vi "Write SerDes GPIO Bank Output Enable.vi"(0 "gpio bank output enable":T2, 2 "serdes id":T1=enum."SI 0 Deserializer") -> (4 "serdes id valid":bool)   [LabVIEW 2020, in "GettingStarted_Common_148X_FPGA.lvlib"]
uses:
  GettingStarted_Common_148X_FPGA.lvlib
  <instrlib>/FlexRIO/CSI-2/v2/FPGA/Types/GPIO Bank.ctl
  Types/SerDes Identifier.ctl
  <vilib>/eio/EIONode/EIONode.xnode
  <vilib>/rvi/eio/common/nirviEmuTemplateMethod_errors.vi
  <instrlib>/_niInstr/Basic Elements/v1/FPGA/niInstr Basic Elements v1 FPGA.lvlib
  <instrlib>/FlexRIO/CSI-2/v2/FPGA/NI CSI-2 API FPGA v2.lvlib
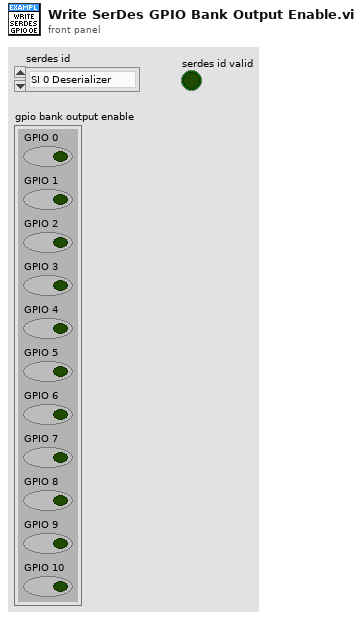
[diagram p1: front panel]
types:
  T1 = typedef "GettingStarted_Common_148X_FPGA.lvlib/SerDes Identifier.ctl" = enum8{"None", "SI 0 Deserializer", "SI 1 Deserializer", "SI 2 Deserializer", "SI 3 Deserializer", "SI 4 Deserializer", "SI 5 Deserializer", "SI 6 Deserializer", "SI 7 Deserializer", "SO 0 Serializer", "SO 1 Serializer", "SO 2 Serializer", "SO 3 Serializer", "SO 4 Serializer", "SO 5 Serializer", "SO 6 Serializer", "SO 7 Serializer", "SI 0 SI 1 Deserializer", "SI 2 SI 3 Deserializer", "SI 4 SI 5 Deserializer", "SI 6 SI 7 Deserializer"}
  T2 = typedef "NI CSI-2 API FPGA v2.lvlib/GPIO Bank.ctl" = cluster{"GPIO 0":bool, "GPIO 1":bool, "GPIO 2":bool, "GPIO 3":bool, "GPIO 4":bool, "GPIO 5":bool, "GPIO 6":bool, "GPIO 7":bool, "GPIO 8":bool, "GPIO 9":bool, "GPIO 10":bool}
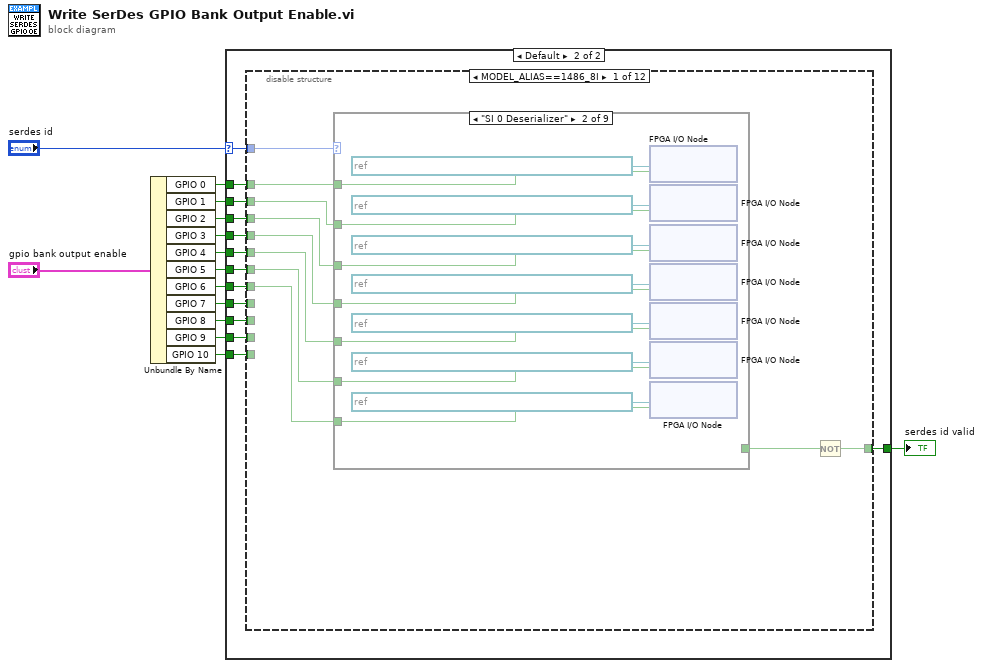
[diagram p0: block diagram]
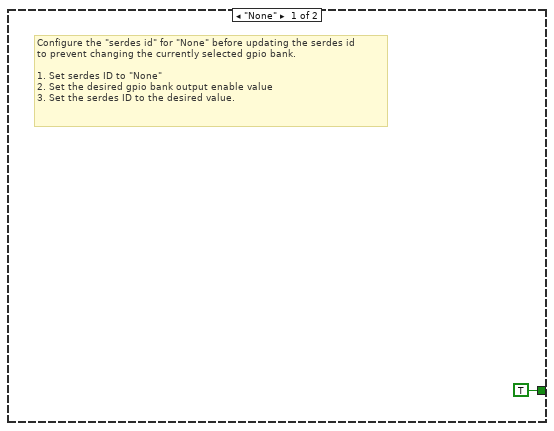
[diagram p2: hidden frame]
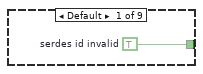
[diagram p3: hidden frame]
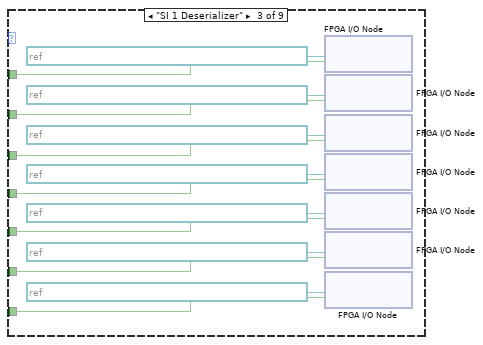
[diagram p4: hidden frame]
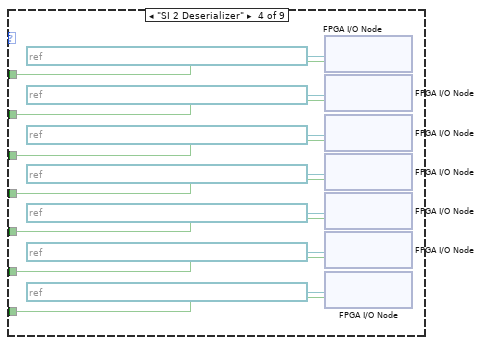
[diagram p5: hidden frame]
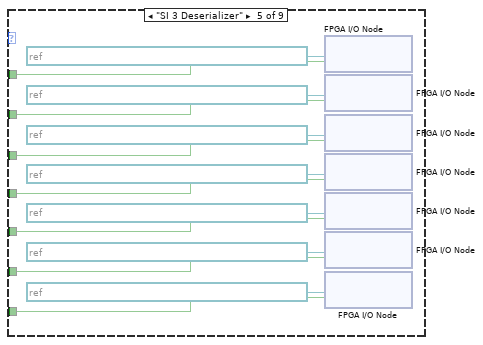
[diagram p6: hidden frame]
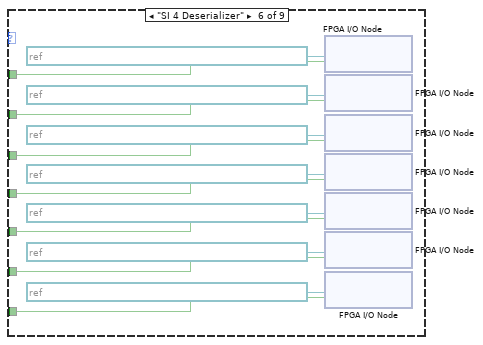
[diagram p7: hidden frame]
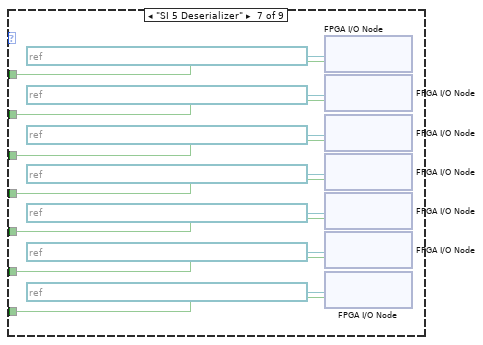
[diagram p8: hidden frame]
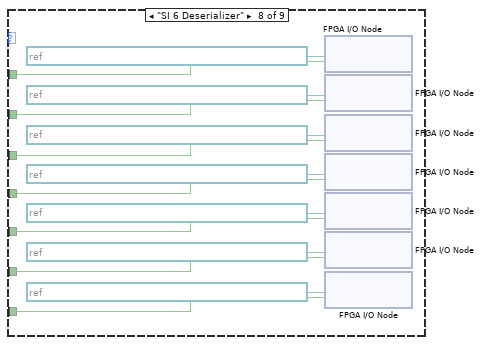
[diagram p9: hidden frame]
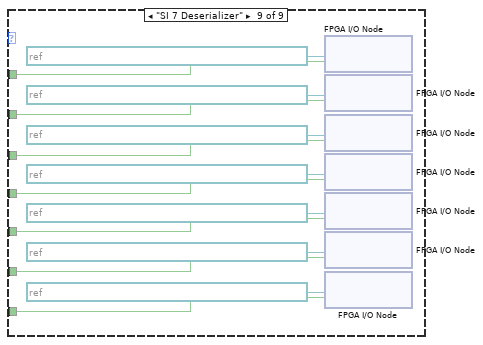
[diagram p10: hidden frame]
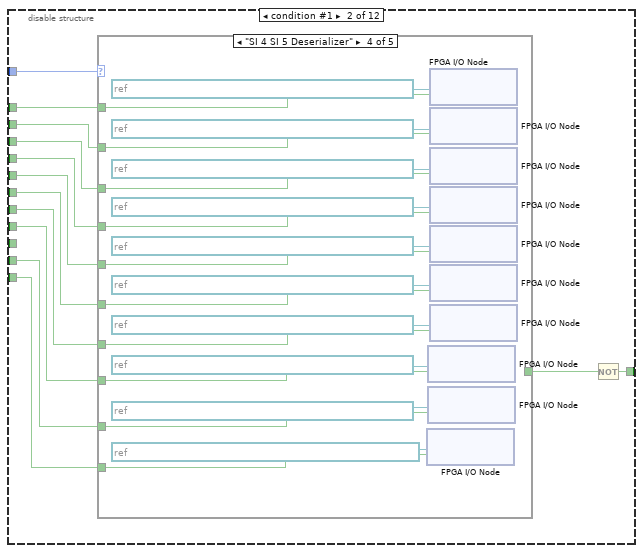
[diagram p11: hidden frame]
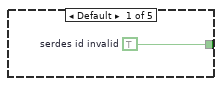
[diagram p12: hidden frame]
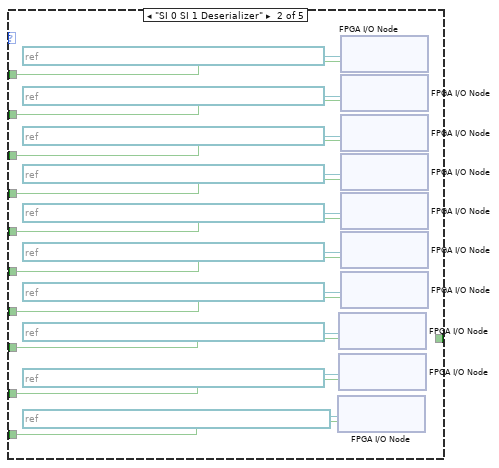
[diagram p13: hidden frame]
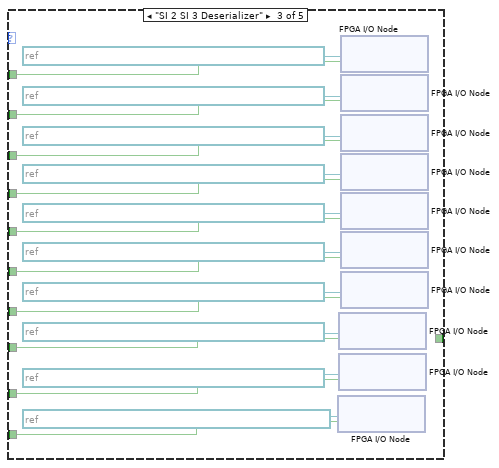
[diagram p14: hidden frame]
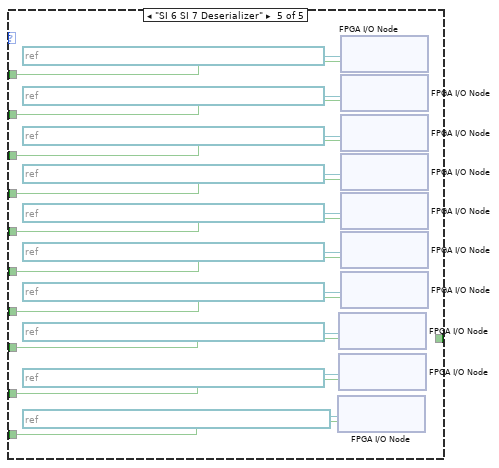
[diagram p15: hidden frame]
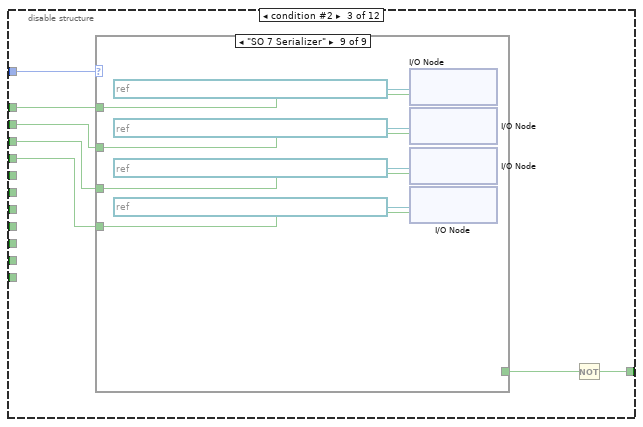
[diagram p16: hidden frame]
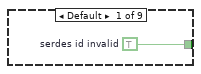
[diagram p17: hidden frame]
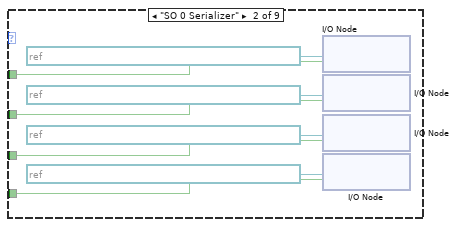
[diagram p18: hidden frame]
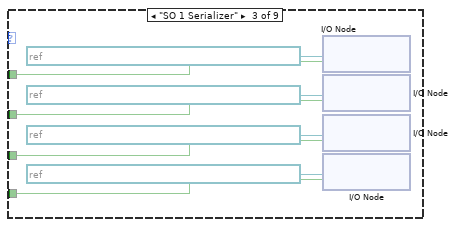
[diagram p19: hidden frame]
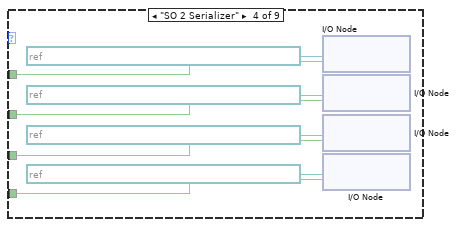
[diagram p20: hidden frame]
diagram:
  n1 = Unbundle By Name("gpio bank output enable") -> ("GPIO 0"=w2:bool, "GPIO 1"=w3:bool, "GPIO 2"=w4:bool, "GPIO 3"=w5:bool, "GPIO 4"=w6:bool, "GPIO 5"=w7:bool, "GPIO 6"=w8:bool, "GPIO 7"=w9:bool, "GPIO 8"=w10:bool, "GPIO 9"=w11:bool, "GPIO 10"=w12:bool)
  n2 = case shown="Default" "serdes id" {
    selector: "serdes id" -> [_ w16]
    tunnel: [TRUE w28] -> w13
    tunnel: w12 -> [_ w27]
    tunnel: w11 -> [_ w26]
    tunnel: w10 -> [_ w25]
    tunnel: w9 -> [_ w24]
    tunnel: w8 -> [_ w23]
    tunnel: w7 -> [_ w22]
    tunnel: w6 -> [_ w21]
    tunnel: w5 -> [_ w20]
    tunnel: w4 -> [_ w19]
    tunnel: w3 -> [_ w18]
    tunnel: w2 -> [_ w17]
    frame "None" {
      # "Configure the \"serdes id\" for \"None\" before updating the serdes id\nto prevent changing the currently selected gpio bank.\n\n1. Set serdes ID to \"None\" \n2. Set the desired gpio bank output enable value \n3. Set the serdes ID to the desired value."
    }
    frame Default {
      n3 = disable-structure shown="MODEL_ALIAS==1486_8I" {
        disable-tunnel: w16 -> [w38 w163 w252 w327 w429 w556 w643 w689 w795 w858 w993 _]
        disable-tunnel: w17 -> [w37 w162 w251 w326 w428 w555 w642 w688 w794 w857 w992 _]
        disable-tunnel: w18 -> [w36 w161 w250 w325 w427 w554 w641 _ _ w856 w991 _]
        disable-tunnel: w19 -> [w35 w160 w249 w324 w426 w553 w640 _ _ w855 w990 _]
        disable-tunnel: w20 -> [w34 w159 w248 w323 w425 w552 w639 w687 w793 w854 w989 _]
        disable-tunnel: w21 -> [w33 w158 _ w322 w424 w551 w638 w686 w792 w853 w988 _]
        disable-tunnel: w22 -> [w32 w157 _ w321 w423 w550 w637 _ _ w852 w987 _]
        disable-tunnel: w23 -> [w31 w156 _ w320 w422 w549 w636 w685 w791 w851 w986 _]
        disable-tunnel: w24 -> [_ w155 _ _ w419 w546 w633 w682 w788 w848 w983 _]
        disable-tunnel: w25 -> [_ _ _ _ _ w545 w632 w681 w787 w847 w982 _]
        disable-tunnel: w26 -> [_ w154 _ _ w418 w544 w631 _ _ w846 w981 _]
        disable-tunnel: w27 -> [_ w153 _ _ w417 w543 w630 _ _ w845 w980 _]
        disable-tunnel: [w29 w164 w246 w318 w420 w547 w634 w683 w789 w849 w984 _] -> w28
        frame condition #0 {
          n4 = case shown="\"SI 0 Deserializer\"" w38 {
            tunnel: w37 -> [_ w46 w60 w74 w88 w102 w116 w130 w144]
            tunnel: w36 -> [_ w45 w59 w73 w87 w101 w115 w129 w143]
            tunnel: w35 -> [_ w44 w58 w72 w86 w100 w114 w128 w142]
            tunnel: w34 -> [_ w43 w57 w71 w85 w99 w113 w127 w141]
            tunnel: w33 -> [_ w42 w56 w70 w84 w98 w112 w126 w140]
            tunnel: w32 -> [_ w41 w55 w69 w83 w97 w111 w125 w139]
            tunnel: w31 -> [_ w40 w54 w68 w82 w96 w110 w124 w138]
            tunnel: [w39 _ _ _ _ _ _ _ _] -> w30
            frame Default {
              w39 = TRUE  # serdes id invalid
            }
            frame "SI 0 Deserializer" {
              n5 = xnode "FPGA I/O Node"("I/O Item"=w46, "FPGA I/O In"=refnum<k21> "IO Socket\\SI 0 Deserializer GPIO 0 Output Enable") -> ()  [unwired: 1 out]
              n6 = xnode "FPGA I/O Node"("I/O Item"=w45, "FPGA I/O In"=refnum<k21> "IO Socket\\SI 0 Deserializer GPIO 1 Output Enable") -> ()  [unwired: 1 out]
              n7 = xnode "FPGA I/O Node"("I/O Item"=w44, "FPGA I/O In"=refnum<k21> "IO Socket\\SI 0 Deserializer GPIO 2 Output Enable") -> ()  [unwired: 1 out]
              n8 = xnode "FPGA I/O Node"("I/O Item"=w43, "FPGA I/O In"=refnum<k21> "IO Socket\\SI 0 Deserializer GPIO 3 Output Enable") -> ()  [unwired: 1 out]
              n9 = xnode "FPGA I/O Node"("I/O Item"=w42, "FPGA I/O In"=refnum<k21> "IO Socket\\SI 0 Deserializer GPIO 4 Output Enable") -> ()  [unwired: 1 out]
              n10 = xnode "FPGA I/O Node"("I/O Item"=w41, "FPGA I/O In"=refnum<k21> "IO Socket\\SI 0 Deserializer GPIO 5 Output Enable") -> ()  [unwired: 1 out]
              n11 = xnode "FPGA I/O Node"("I/O Item"=w40, "FPGA I/O In"=refnum<k21> "IO Socket\\SI 0 Deserializer GPIO 6 Output Enable") -> ()  [unwired: 1 out]
            }
            frame "SI 1 Deserializer" {
              n12 = xnode "FPGA I/O Node"("I/O Item"=w60, "FPGA I/O In"=refnum<k21> "IO Socket\\SI 1 Deserializer GPIO 0 Output Enable") -> ()  [unwired: 1 out]
              n13 = xnode "FPGA I/O Node"("I/O Item"=w59, "FPGA I/O In"=refnum<k21> "IO Socket\\SI 1 Deserializer GPIO 1 Output Enable") -> ()  [unwired: 1 out]
              n14 = xnode "FPGA I/O Node"("I/O Item"=w58, "FPGA I/O In"=refnum<k21> "IO Socket\\SI 1 Deserializer GPIO 2 Output Enable") -> ()  [unwired: 1 out]
              n15 = xnode "FPGA I/O Node"("I/O Item"=w57, "FPGA I/O In"=refnum<k21> "IO Socket\\SI 1 Deserializer GPIO 3 Output Enable") -> ()  [unwired: 1 out]
              n16 = xnode "FPGA I/O Node"("I/O Item"=w56, "FPGA I/O In"=refnum<k21> "IO Socket\\SI 1 Deserializer GPIO 4 Output Enable") -> ()  [unwired: 1 out]
              n17 = xnode "FPGA I/O Node"("I/O Item"=w55, "FPGA I/O In"=refnum<k21> "IO Socket\\SI 1 Deserializer GPIO 5 Output Enable") -> ()  [unwired: 1 out]
              n18 = xnode "FPGA I/O Node"("I/O Item"=w54, "FPGA I/O In"=refnum<k21> "IO Socket\\SI 1 Deserializer GPIO 6 Output Enable") -> ()  [unwired: 1 out]
            }
            frame "SI 2 Deserializer" {
              n19 = xnode "FPGA I/O Node"("I/O Item"=w74, "FPGA I/O In"=refnum<k21> "IO Socket\\SI 2 Deserializer GPIO 0 Output Enable") -> ()  [unwired: 1 out]
              n20 = xnode "FPGA I/O Node"("I/O Item"=w73, "FPGA I/O In"=refnum<k21> "IO Socket\\SI 2 Deserializer GPIO 1 Output Enable") -> ()  [unwired: 1 out]
              n21 = xnode "FPGA I/O Node"("I/O Item"=w72, "FPGA I/O In"=refnum<k21> "IO Socket\\SI 2 Deserializer GPIO 2 Output Enable") -> ()  [unwired: 1 out]
              n22 = xnode "FPGA I/O Node"("I/O Item"=w71, "FPGA I/O In"=refnum<k21> "IO Socket\\SI 2 Deserializer GPIO 3 Output Enable") -> ()  [unwired: 1 out]
              n23 = xnode "FPGA I/O Node"("I/O Item"=w70, "FPGA I/O In"=refnum<k21> "IO Socket\\SI 2 Deserializer GPIO 4 Output Enable") -> ()  [unwired: 1 out]
              n24 = xnode "FPGA I/O Node"("I/O Item"=w69, "FPGA I/O In"=refnum<k21> "IO Socket\\SI 2 Deserializer GPIO 5 Output Enable") -> ()  [unwired: 1 out]
              n25 = xnode "FPGA I/O Node"("I/O Item"=w68, "FPGA I/O In"=refnum<k21> "IO Socket\\SI 2 Deserializer GPIO 6 Output Enable") -> ()  [unwired: 1 out]
            }
            frame "SI 3 Deserializer" {
              n26 = xnode "FPGA I/O Node"("I/O Item"=w88, "FPGA I/O In"=refnum<k21> "IO Socket\\SI 3 Deserializer GPIO 0 Output Enable") -> ()  [unwired: 1 out]
              n27 = xnode "FPGA I/O Node"("I/O Item"=w87, "FPGA I/O In"=refnum<k21> "IO Socket\\SI 3 Deserializer GPIO 1 Output Enable") -> ()  [unwired: 1 out]
              n28 = xnode "FPGA I/O Node"("I/O Item"=w86, "FPGA I/O In"=refnum<k21> "IO Socket\\SI 3 Deserializer GPIO 2 Output Enable") -> ()  [unwired: 1 out]
              n29 = xnode "FPGA I/O Node"("I/O Item"=w85, "FPGA I/O In"=refnum<k21> "IO Socket\\SI 3 Deserializer GPIO 3 Output Enable") -> ()  [unwired: 1 out]
              n30 = xnode "FPGA I/O Node"("I/O Item"=w84, "FPGA I/O In"=refnum<k21> "IO Socket\\SI 3 Deserializer GPIO 4 Output Enable") -> ()  [unwired: 1 out]
              n31 = xnode "FPGA I/O Node"("I/O Item"=w83, "FPGA I/O In"=refnum<k21> "IO Socket\\SI 3 Deserializer GPIO 5 Output Enable") -> ()  [unwired: 1 out]
              n32 = xnode "FPGA I/O Node"("I/O Item"=w82, "FPGA I/O In"=refnum<k21> "IO Socket\\SI 3 Deserializer GPIO 6 Output Enable") -> ()  [unwired: 1 out]
            }
            frame "SI 4 Deserializer" {
              n33 = xnode "FPGA I/O Node"("I/O Item"=w102, "FPGA I/O In"=refnum<k21> "IO Socket\\SI 4 Deserializer GPIO 0 Output Enable") -> ()  [unwired: 1 out]
              n34 = xnode "FPGA I/O Node"("I/O Item"=w101, "FPGA I/O In"=refnum<k21> "IO Socket\\SI 4 Deserializer GPIO 1 Output Enable") -> ()  [unwired: 1 out]
              n35 = xnode "FPGA I/O Node"("I/O Item"=w100, "FPGA I/O In"=refnum<k21> "IO Socket\\SI 4 Deserializer GPIO 2 Output Enable") -> ()  [unwired: 1 out]
              n36 = xnode "FPGA I/O Node"("I/O Item"=w99, "FPGA I/O In"=refnum<k21> "IO Socket\\SI 4 Deserializer GPIO 3 Output Enable") -> ()  [unwired: 1 out]
              n37 = xnode "FPGA I/O Node"("I/O Item"=w98, "FPGA I/O In"=refnum<k21> "IO Socket\\SI 4 Deserializer GPIO 4 Output Enable") -> ()  [unwired: 1 out]
              n38 = xnode "FPGA I/O Node"("I/O Item"=w97, "FPGA I/O In"=refnum<k21> "IO Socket\\SI 4 Deserializer GPIO 5 Output Enable") -> ()  [unwired: 1 out]
              n39 = xnode "FPGA I/O Node"("I/O Item"=w96, "FPGA I/O In"=refnum<k21> "IO Socket\\SI 4 Deserializer GPIO 6 Output Enable") -> ()  [unwired: 1 out]
            }
            frame "SI 5 Deserializer" {
              n40 = xnode "FPGA I/O Node"("I/O Item"=w116, "FPGA I/O In"=refnum<k21> "IO Socket\\SI 5 Deserializer GPIO 0 Output Enable") -> ()  [unwired: 1 out]
              n41 = xnode "FPGA I/O Node"("I/O Item"=w115, "FPGA I/O In"=refnum<k21> "IO Socket\\SI 5 Deserializer GPIO 1 Output Enable") -> ()  [unwired: 1 out]
              n42 = xnode "FPGA I/O Node"("I/O Item"=w114, "FPGA I/O In"=refnum<k21> "IO Socket\\SI 5 Deserializer GPIO 2 Output Enable") -> ()  [unwired: 1 out]
              n43 = xnode "FPGA I/O Node"("I/O Item"=w113, "FPGA I/O In"=refnum<k21> "IO Socket\\SI 5 Deserializer GPIO 3 Output Enable") -> ()  [unwired: 1 out]
              n44 = xnode "FPGA I/O Node"("I/O Item"=w112, "FPGA I/O In"=refnum<k21> "IO Socket\\SI 5 Deserializer GPIO 4 Output Enable") -> ()  [unwired: 1 out]
              n45 = xnode "FPGA I/O Node"("I/O Item"=w111, "FPGA I/O In"=refnum<k21> "IO Socket\\SI 5 Deserializer GPIO 5 Output Enable") -> ()  [unwired: 1 out]
              n46 = xnode "FPGA I/O Node"("I/O Item"=w110, "FPGA I/O In"=refnum<k21> "IO Socket\\SI 5 Deserializer GPIO 6 Output Enable") -> ()  [unwired: 1 out]
            }
            frame "SI 6 Deserializer" {
              n47 = xnode "FPGA I/O Node"("I/O Item"=w130, "FPGA I/O In"=refnum<k21> "IO Socket\\SI 6 Deserializer GPIO 0 Output Enable") -> ()  [unwired: 1 out]
              n48 = xnode "FPGA I/O Node"("I/O Item"=w129, "FPGA I/O In"=refnum<k21> "IO Socket\\SI 6 Deserializer GPIO 1 Output Enable") -> ()  [unwired: 1 out]
              n49 = xnode "FPGA I/O Node"("I/O Item"=w128, "FPGA I/O In"=refnum<k21> "IO Socket\\SI 6 Deserializer GPIO 2 Output Enable") -> ()  [unwired: 1 out]
              n50 = xnode "FPGA I/O Node"("I/O Item"=w127, "FPGA I/O In"=refnum<k21> "IO Socket\\SI 6 Deserializer GPIO 3 Output Enable") -> ()  [unwired: 1 out]
              n51 = xnode "FPGA I/O Node"("I/O Item"=w126, "FPGA I/O In"=refnum<k21> "IO Socket\\SI 6 Deserializer GPIO 4 Output Enable") -> ()  [unwired: 1 out]
              n52 = xnode "FPGA I/O Node"("I/O Item"=w125, "FPGA I/O In"=refnum<k21> "IO Socket\\SI 6 Deserializer GPIO 5 Output Enable") -> ()  [unwired: 1 out]
              n53 = xnode "FPGA I/O Node"("I/O Item"=w124, "FPGA I/O In"=refnum<k21> "IO Socket\\SI 6 Deserializer GPIO 6 Output Enable") -> ()  [unwired: 1 out]
            }
            frame "SI 7 Deserializer" {
              n54 = xnode "FPGA I/O Node"("I/O Item"=w144, "FPGA I/O In"=refnum<k21> "IO Socket\\SI 7 Deserializer GPIO 0 Output Enable") -> ()  [unwired: 1 out]
              n55 = xnode "FPGA I/O Node"("I/O Item"=w143, "FPGA I/O In"=refnum<k21> "IO Socket\\SI 7 Deserializer GPIO 1 Output Enable") -> ()  [unwired: 1 out]
              n56 = xnode "FPGA I/O Node"("I/O Item"=w142, "FPGA I/O In"=refnum<k21> "IO Socket\\SI 7 Deserializer GPIO 2 Output Enable") -> ()  [unwired: 1 out]
              n57 = xnode "FPGA I/O Node"("I/O Item"=w141, "FPGA I/O In"=refnum<k21> "IO Socket\\SI 7 Deserializer GPIO 3 Output Enable") -> ()  [unwired: 1 out]
              n58 = xnode "FPGA I/O Node"("I/O Item"=w140, "FPGA I/O In"=refnum<k21> "IO Socket\\SI 7 Deserializer GPIO 4 Output Enable") -> ()  [unwired: 1 out]
              n59 = xnode "FPGA I/O Node"("I/O Item"=w139, "FPGA I/O In"=refnum<k21> "IO Socket\\SI 7 Deserializer GPIO 5 Output Enable") -> ()  [unwired: 1 out]
              n60 = xnode "FPGA I/O Node"("I/O Item"=w138, "FPGA I/O In"=refnum<k21> "IO Socket\\SI 7 Deserializer GPIO 6 Output Enable") -> ()  [unwired: 1 out]
            }
          }
          n61 = Not(x=w30) -> (.not. x?=w29:bool)
        }
        frame condition #1 {
          n62 = case shown="\"SI 4 SI 5 Deserializer\"" w163 {
            tunnel: w162 -> [_ w185 w205 w225 w245]
            tunnel: w161 -> [_ w184 w204 w224 w244]
            tunnel: w160 -> [_ w183 w203 w223 w243]
            tunnel: w159 -> [_ w182 w202 w222 w242]
            tunnel: w158 -> [_ w181 w201 w221 w241]
            tunnel: w157 -> [_ w180 w200 w220 w240]
            tunnel: w156 -> [_ w179 w199 w219 w239]
            tunnel: [w165 _ _ _ _] -> w152
            tunnel: w155 -> [_ w168 w188 w208 w228]
            tunnel: w154 -> [_ w167 w187 w207 w227]
            tunnel: w153 -> [_ w166 w186 w206 w226]
            frame Default {
              w165 = TRUE  # serdes id invalid
            }
            frame "SI 0 SI 1 Deserializer" {
              n63 = xnode "FPGA I/O Node"("I/O Item"=w166, "FPGA I/O In"=refnum<k21> "IO Socket\\SI 0 SI 1 Deserializer GPIO 10 Output Enable") -> ()  [unwired: 1 out]
              n64 = xnode "FPGA I/O Node"("I/O Item"=w168, "FPGA I/O In"=refnum<k21> "IO Socket\\SI 0 SI 1 Deserializer GPIO 7 Output Enable") -> ()  [unwired: 1 out]
              n65 = xnode "FPGA I/O Node"("I/O Item"=w167, "FPGA I/O In"=refnum<k21> "IO Socket\\SI 0 SI 1 Deserializer GPIO 9 Output Enable") -> ()  [unwired: 1 out]
              n66 = xnode "FPGA I/O Node"("I/O Item"=w185, "FPGA I/O In"=refnum<k21> "IO Socket\\SI 0 SI 1 Deserializer GPIO 0 Output Enable") -> ()  [unwired: 1 out]
              n67 = xnode "FPGA I/O Node"("I/O Item"=w184, "FPGA I/O In"=refnum<k21> "IO Socket\\SI 0 SI 1 Deserializer GPIO 1 Output Enable") -> ()  [unwired: 1 out]
              n68 = xnode "FPGA I/O Node"("I/O Item"=w183, "FPGA I/O In"=refnum<k21> "IO Socket\\SI 0 SI 1 Deserializer GPIO 2 Output Enable") -> ()  [unwired: 1 out]
              n69 = xnode "FPGA I/O Node"("I/O Item"=w182, "FPGA I/O In"=refnum<k21> "IO Socket\\SI 0 SI 1 Deserializer GPIO 3 Output Enable") -> ()  [unwired: 1 out]
              n70 = xnode "FPGA I/O Node"("I/O Item"=w181, "FPGA I/O In"=refnum<k21> "IO Socket\\SI 0 SI 1 Deserializer GPIO 4 Output Enable") -> ()  [unwired: 1 out]
              n71 = xnode "FPGA I/O Node"("I/O Item"=w180, "FPGA I/O In"=refnum<k21> "IO Socket\\SI 0 SI 1 Deserializer GPIO 5 Output Enable") -> ()  [unwired: 1 out]
              n72 = xnode "FPGA I/O Node"("I/O Item"=w179, "FPGA I/O In"=refnum<k21> "IO Socket\\SI 0 SI 1 Deserializer GPIO 6 Output Enable") -> ()  [unwired: 1 out]
            }
            frame "SI 2 SI 3 Deserializer" {
              n73 = xnode "FPGA I/O Node"("I/O Item"=w186, "FPGA I/O In"=refnum<k21> "IO Socket\\SI 2 SI 3 Deserializer GPIO 10 Output Enable") -> ()  [unwired: 1 out]
              n74 = xnode "FPGA I/O Node"("I/O Item"=w188, "FPGA I/O In"=refnum<k21> "IO Socket\\SI 2 SI 3 Deserializer GPIO 7 Output Enable") -> ()  [unwired: 1 out]
              n75 = xnode "FPGA I/O Node"("I/O Item"=w187, "FPGA I/O In"=refnum<k21> "IO Socket\\SI 2 SI 3 Deserializer GPIO 9 Output Enable") -> ()  [unwired: 1 out]
              n76 = xnode "FPGA I/O Node"("I/O Item"=w205, "FPGA I/O In"=refnum<k21> "IO Socket\\SI 2 SI 3 Deserializer GPIO 0 Output Enable") -> ()  [unwired: 1 out]
              n77 = xnode "FPGA I/O Node"("I/O Item"=w204, "FPGA I/O In"=refnum<k21> "IO Socket\\SI 2 SI 3 Deserializer GPIO 1 Output Enable") -> ()  [unwired: 1 out]
              n78 = xnode "FPGA I/O Node"("I/O Item"=w203, "FPGA I/O In"=refnum<k21> "IO Socket\\SI 2 SI 3 Deserializer GPIO 2 Output Enable") -> ()  [unwired: 1 out]
              n79 = xnode "FPGA I/O Node"("I/O Item"=w202, "FPGA I/O In"=refnum<k21> "IO Socket\\SI 2 SI 3 Deserializer GPIO 3 Output Enable") -> ()  [unwired: 1 out]
              n80 = xnode "FPGA I/O Node"("I/O Item"=w201, "FPGA I/O In"=refnum<k21> "IO Socket\\SI 2 SI 3 Deserializer GPIO 4 Output Enable") -> ()  [unwired: 1 out]
              n81 = xnode "FPGA I/O Node"("I/O Item"=w200, "FPGA I/O In"=refnum<k21> "IO Socket\\SI 2 SI 3 Deserializer GPIO 5 Output Enable") -> ()  [unwired: 1 out]
              n82 = xnode "FPGA I/O Node"("I/O Item"=w199, "FPGA I/O In"=refnum<k21> "IO Socket\\SI 2 SI 3 Deserializer GPIO 6 Output Enable") -> ()  [unwired: 1 out]
            }
            frame "SI 4 SI 5 Deserializer" {
              n83 = xnode "FPGA I/O Node"("I/O Item"=w206, "FPGA I/O In"=refnum<k21> "IO Socket\\SI 4 SI 5 Deserializer GPIO 10 Output Enable") -> ()  [unwired: 1 out]
              n84 = xnode "FPGA I/O Node"("I/O Item"=w208, "FPGA I/O In"=refnum<k21> "IO Socket\\SI 4 SI 5 Deserializer GPIO 7 Output Enable") -> ()  [unwired: 1 out]
              n85 = xnode "FPGA I/O Node"("I/O Item"=w207, "FPGA I/O In"=refnum<k21> "IO Socket\\SI 4 SI 5 Deserializer GPIO 9 Output Enable") -> ()  [unwired: 1 out]
              n86 = xnode "FPGA I/O Node"("I/O Item"=w225, "FPGA I/O In"=refnum<k21> "IO Socket\\SI 4 SI 5 Deserializer GPIO 0 Output Enable") -> ()  [unwired: 1 out]
              n87 = xnode "FPGA I/O Node"("I/O Item"=w224, "FPGA I/O In"=refnum<k21> "IO Socket\\SI 4 SI 5 Deserializer GPIO 1 Output Enable") -> ()  [unwired: 1 out]
              n88 = xnode "FPGA I/O Node"("I/O Item"=w223, "FPGA I/O In"=refnum<k21> "IO Socket\\SI 4 SI 5 Deserializer GPIO 2 Output Enable") -> ()  [unwired: 1 out]
              n89 = xnode "FPGA I/O Node"("I/O Item"=w222, "FPGA I/O In"=refnum<k21> "IO Socket\\SI 4 SI 5 Deserializer GPIO 3 Output Enable") -> ()  [unwired: 1 out]
              n90 = xnode "FPGA I/O Node"("I/O Item"=w221, "FPGA I/O In"=refnum<k21> "IO Socket\\SI 4 SI 5 Deserializer GPIO 4 Output Enable") -> ()  [unwired: 1 out]
              n91 = xnode "FPGA I/O Node"("I/O Item"=w220, "FPGA I/O In"=refnum<k21> "IO Socket\\SI 4 SI 5 Deserializer GPIO 5 Output Enable") -> ()  [unwired: 1 out]
              n92 = xnode "FPGA I/O Node"("I/O Item"=w219, "FPGA I/O In"=refnum<k21> "IO Socket\\SI 4 SI 5 Deserializer GPIO 6 Output Enable") -> ()  [unwired: 1 out]
            }
            frame "SI 6 SI 7 Deserializer" {
              n93 = xnode "FPGA I/O Node"("I/O Item"=w226, "FPGA I/O In"=refnum<k21> "IO Socket\\SI 6 SI 7 Deserializer GPIO 10 Output Enable") -> ()  [unwired: 1 out]
              n94 = xnode "FPGA I/O Node"("I/O Item"=w228, "FPGA I/O In"=refnum<k21> "IO Socket\\SI 6 SI 7 Deserializer GPIO 7 Output Enable") -> ()  [unwired: 1 out]
              n95 = xnode "FPGA I/O Node"("I/O Item"=w227, "FPGA I/O In"=refnum<k21> "IO Socket\\SI 6 SI 7 Deserializer GPIO 9 Output Enable") -> ()  [unwired: 1 out]
              n96 = xnode "FPGA I/O Node"("I/O Item"=w245, "FPGA I/O In"=refnum<k21> "IO Socket\\SI 6 SI 7 Deserializer GPIO 0 Output Enable") -> ()  [unwired: 1 out]
              n97 = xnode "FPGA I/O Node"("I/O Item"=w244, "FPGA I/O In"=refnum<k21> "IO Socket\\SI 6 SI 7 Deserializer GPIO 1 Output Enable") -> ()  [unwired: 1 out]
              n98 = xnode "FPGA I/O Node"("I/O Item"=w243, "FPGA I/O In"=refnum<k21> "IO Socket\\SI 6 SI 7 Deserializer GPIO 2 Output Enable") -> ()  [unwired: 1 out]
              n99 = xnode "FPGA I/O Node"("I/O Item"=w242, "FPGA I/O In"=refnum<k21> "IO Socket\\SI 6 SI 7 Deserializer GPIO 3 Output Enable") -> ()  [unwired: 1 out]
              n100 = xnode "FPGA I/O Node"("I/O Item"=w241, "FPGA I/O In"=refnum<k21> "IO Socket\\SI 6 SI 7 Deserializer GPIO 4 Output Enable") -> ()  [unwired: 1 out]
              n101 = xnode "FPGA I/O Node"("I/O Item"=w240, "FPGA I/O In"=refnum<k21> "IO Socket\\SI 6 SI 7 Deserializer GPIO 5 Output Enable") -> ()  [unwired: 1 out]
              n102 = xnode "FPGA I/O Node"("I/O Item"=w239, "FPGA I/O In"=refnum<k21> "IO Socket\\SI 6 SI 7 Deserializer GPIO 6 Output Enable") -> ()  [unwired: 1 out]
            }
          }
          n103 = Not(x=w152) -> (.not. x?=w164:bool)
        }
        frame condition #2 {
          n104 = case shown="\"SO 7 Serializer\"" w252 {
            tunnel: w251 -> [_ w257 w265 w273 w281 w289 w297 w305 w313]
            tunnel: w250 -> [_ w256 w264 w272 w280 w288 w296 w304 w312]
            tunnel: w249 -> [_ w255 w263 w271 w279 w287 w295 w303 w311]
            tunnel: w248 -> [_ w254 w262 w270 w278 w286 w294 w302 w310]
            tunnel: [w253 _ _ _ _ _ _ _ _] -> w247
            frame Default {
              w253 = TRUE  # serdes id invalid
            }
            frame "SO 0 Serializer" {
              n105 = xnode "I/O Node"("I/O Item"=w257, "FPGA I/O In"=refnum<k21> "IO Socket\\SO 0 Serializer GPIO 0 Output Enable") -> ()  [unwired: 1 out]
              n106 = xnode "I/O Node"("I/O Item"=w256, "FPGA I/O In"=refnum<k21> "IO Socket\\SO 0 Serializer GPIO 1 Output Enable") -> ()  [unwired: 1 out]
              n107 = xnode "I/O Node"("I/O Item"=w255, "FPGA I/O In"=refnum<k21> "IO Socket\\SO 0 Serializer GPIO 2 Output Enable") -> ()  [unwired: 1 out]
              n108 = xnode "I/O Node"("I/O Item"=w254, "FPGA I/O In"=refnum<k21> "IO Socket\\SO 0 Serializer GPIO 3 Output Enable") -> ()  [unwired: 1 out]
            }
            frame "SO 1 Serializer" {
              n109 = xnode "I/O Node"("I/O Item"=w265, "FPGA I/O In"=refnum<k21> "IO Socket\\SO 1 Serializer GPIO 0 Output Enable") -> ()  [unwired: 1 out]
              n110 = xnode "I/O Node"("I/O Item"=w264, "FPGA I/O In"=refnum<k21> "IO Socket\\SO 1 Serializer GPIO 1 Output Enable") -> ()  [unwired: 1 out]
              n111 = xnode "I/O Node"("I/O Item"=w263, "FPGA I/O In"=refnum<k21> "IO Socket\\SO 1 Serializer GPIO 2 Output Enable") -> ()  [unwired: 1 out]
              n112 = xnode "I/O Node"("I/O Item"=w262, "FPGA I/O In"=refnum<k21> "IO Socket\\SO 1 Serializer GPIO 3 Output Enable") -> ()  [unwired: 1 out]
            }
            frame "SO 2 Serializer" {
              n113 = xnode "I/O Node"("I/O Item"=w273, "FPGA I/O In"=refnum<k21> "IO Socket\\SO 2 Serializer GPIO 0 Output Enable") -> ()  [unwired: 1 out]
              n114 = xnode "I/O Node"("I/O Item"=w272, "FPGA I/O In"=refnum<k21> "IO Socket\\SO 2 Serializer GPIO 1 Output Enable") -> ()  [unwired: 1 out]
              n115 = xnode "I/O Node"("I/O Item"=w271, "FPGA I/O In"=refnum<k21> "IO Socket\\SO 2 Serializer GPIO 2 Output Enable") -> ()  [unwired: 1 out]
              n116 = xnode "I/O Node"("I/O Item"=w270, "FPGA I/O In"=refnum<k21> "IO Socket\\SO 2 Serializer GPIO 3 Output Enable") -> ()  [unwired: 1 out]
            }
            frame "SO 3 Serializer" {
              n117 = xnode "I/O Node"("I/O Item"=w281, "FPGA I/O In"=refnum<k21> "IO Socket\\SO 3 Serializer GPIO 0 Output Enable") -> ()  [unwired: 1 out]
              n118 = xnode "I/O Node"("I/O Item"=w280, "FPGA I/O In"=refnum<k21> "IO Socket\\SO 3 Serializer GPIO 1 Output Enable") -> ()  [unwired: 1 out]
              n119 = xnode "I/O Node"("I/O Item"=w279, "FPGA I/O In"=refnum<k21> "IO Socket\\SO 3 Serializer GPIO 2 Output Enable") -> ()  [unwired: 1 out]
              n120 = xnode "I/O Node"("I/O Item"=w278, "FPGA I/O In"=refnum<k21> "IO Socket\\SO 3 Serializer GPIO 3 Output Enable") -> ()  [unwired: 1 out]
            }
            frame "SO 4 Serializer" {
              n121 = xnode "I/O Node"("I/O Item"=w289, "FPGA I/O In"=refnum<k21> "IO Socket\\SO 4 Serializer GPIO 0 Output Enable") -> ()  [unwired: 1 out]
              n122 = xnode "I/O Node"("I/O Item"=w288, "FPGA I/O In"=refnum<k21> "IO Socket\\SO 4 Serializer GPIO 1 Output Enable") -> ()  [unwired: 1 out]
              n123 = xnode "I/O Node"("I/O Item"=w287, "FPGA I/O In"=refnum<k21> "IO Socket\\SO 4 Serializer GPIO 2 Output Enable") -> ()  [unwired: 1 out]
              n124 = xnode "I/O Node"("I/O Item"=w286, "FPGA I/O In"=refnum<k21> "IO Socket\\SO 4 Serializer GPIO 3 Output Enable") -> ()  [unwired: 1 out]
            }
            frame "SO 5 Serializer" {
              n125 = xnode "I/O Node"("I/O Item"=w297, "FPGA I/O In"=refnum<k21> "IO Socket\\SO 5 Serializer GPIO 0 Output Enable") -> ()  [unwired: 1 out]
              n126 = xnode "I/O Node"("I/O Item"=w296, "FPGA I/O In"=refnum<k21> "IO Socket\\SO 5 Serializer GPIO 1 Output Enable") -> ()  [unwired: 1 out]
              n127 = xnode "I/O Node"("I/O Item"=w295, "FPGA I/O In"=refnum<k21> "IO Socket\\SO 5 Serializer GPIO 2 Output Enable") -> ()  [unwired: 1 out]
              n128 = xnode "I/O Node"("I/O Item"=w294, "FPGA I/O In"=refnum<k21> "IO Socket\\SO 5 Serializer GPIO 3 Output Enable") -> ()  [unwired: 1 out]
            }
            frame "SO 6 Serializer" {
              n129 = xnode "I/O Node"("I/O Item"=w305, "FPGA I/O In"=refnum<k21> "IO Socket\\SO 6 Serializer GPIO 0 Output Enable") -> ()  [unwired: 1 out]
              n130 = xnode "I/O Node"("I/O Item"=w304, "FPGA I/O In"=refnum<k21> "IO Socket\\SO 6 Serializer GPIO 1 Output Enable") -> ()  [unwired: 1 out]
              n131 = xnode "I/O Node"("I/O Item"=w303, "FPGA I/O In"=refnum<k21> "IO Socket\\SO 6 Serializer GPIO 2 Output Enable") -> ()  [unwired: 1 out]
              n132 = xnode "I/O Node"("I/O Item"=w302, "FPGA I/O In"=refnum<k21> "IO Socket\\SO 6 Serializer GPIO 3 Output Enable") -> ()  [unwired: 1 out]
            }
            frame "SO 7 Serializer" {
              n133 = xnode "I/O Node"("I/O Item"=w313, "FPGA I/O In"=refnum<k21> "IO Socket\\SO 7 Serializer GPIO 0 Output Enable") -> ()  [unwired: 1 out]
              n134 = xnode "I/O Node"("I/O Item"=w312, "FPGA I/O In"=refnum<k21> "IO Socket\\SO 7 Serializer GPIO 1 Output Enable") -> ()  [unwired: 1 out]
              n135 = xnode "I/O Node"("I/O Item"=w311, "FPGA I/O In"=refnum<k21> "IO Socket\\SO 7 Serializer GPIO 2 Output Enable") -> ()  [unwired: 1 out]
              n136 = xnode "I/O Node"("I/O Item"=w310, "FPGA I/O In"=refnum<k21> "IO Socket\\SO 7 Serializer GPIO 3 Output Enable") -> ()  [unwired: 1 out]
            }
          }
          n137 = Not(x=w247) -> (.not. x?=w246:bool)
        }
        frame condition #3 {
          n138 = case shown="\"SO 1 Serializer\"" w327 {
            tunnel: w326 -> [_ w335 w349 w363 w377 w388 w396 w404 w412]
            tunnel: w325 -> [_ w334 w348 w362 w376 w387 w395 w403 w411]
            tunnel: w324 -> [_ w333 w347 w361 w375 w386 w394 w402 w410]
            tunnel: w323 -> [_ w332 w346 w360 w374 w385 w393 w401 w409]
            tunnel: w322 -> [_ w331 w345 w359 w373 _ _ _ _]
            tunnel: w321 -> [_ w330 w344 w358 w372 _ _ _ _]
            tunnel: w320 -> [_ w329 w343 w357 w371 _ _ _ _]
            tunnel: [w328 _ _ _ _ _ _ _ _] -> w319
            frame Default {
              w328 = TRUE  # serdes id invalid
            }
            frame "SI 0 Deserializer" {
              n139 = xnode "FPGA I/O Node"("I/O Item"=w335, "FPGA I/O In"=refnum<k21> "IO Socket\\SI 0 Deserializer GPIO 0 Output Enable") -> ()  [unwired: 1 out]
              n140 = xnode "FPGA I/O Node"("I/O Item"=w334, "FPGA I/O In"=refnum<k21> "IO Socket\\SI 0 Deserializer GPIO 1 Output Enable") -> ()  [unwired: 1 out]
              n141 = xnode "FPGA I/O Node"("I/O Item"=w333, "FPGA I/O In"=refnum<k21> "IO Socket\\SI 0 Deserializer GPIO 2 Output Enable") -> ()  [unwired: 1 out]
              n142 = xnode "FPGA I/O Node"("I/O Item"=w332, "FPGA I/O In"=refnum<k21> "IO Socket\\SI 0 Deserializer GPIO 3 Output Enable") -> ()  [unwired: 1 out]
              n143 = xnode "FPGA I/O Node"("I/O Item"=w331, "FPGA I/O In"=refnum<k21> "IO Socket\\SI 0 Deserializer GPIO 4 Output Enable") -> ()  [unwired: 1 out]
              n144 = xnode "FPGA I/O Node"("I/O Item"=w330, "FPGA I/O In"=refnum<k21> "IO Socket\\SI 0 Deserializer GPIO 5 Output Enable") -> ()  [unwired: 1 out]
              n145 = xnode "FPGA I/O Node"("I/O Item"=w329, "FPGA I/O In"=refnum<k21> "IO Socket\\SI 0 Deserializer GPIO 6 Output Enable") -> ()  [unwired: 1 out]
            }
            frame "SI 1 Deserializer" {
              n146 = xnode "FPGA I/O Node"("I/O Item"=w349, "FPGA I/O In"=refnum<k21> "IO Socket\\SI 1 Deserializer GPIO 0 Output Enable") -> ()  [unwired: 1 out]
              n147 = xnode "FPGA I/O Node"("I/O Item"=w348, "FPGA I/O In"=refnum<k21> "IO Socket\\SI 1 Deserializer GPIO 1 Output Enable") -> ()  [unwired: 1 out]
              n148 = xnode "FPGA I/O Node"("I/O Item"=w347, "FPGA I/O In"=refnum<k21> "IO Socket\\SI 1 Deserializer GPIO 2 Output Enable") -> ()  [unwired: 1 out]
              n149 = xnode "FPGA I/O Node"("I/O Item"=w346, "FPGA I/O In"=refnum<k21> "IO Socket\\SI 1 Deserializer GPIO 3 Output Enable") -> ()  [unwired: 1 out]
              n150 = xnode "FPGA I/O Node"("I/O Item"=w345, "FPGA I/O In"=refnum<k21> "IO Socket\\SI 1 Deserializer GPIO 4 Output Enable") -> ()  [unwired: 1 out]
              n151 = xnode "FPGA I/O Node"("I/O Item"=w344, "FPGA I/O In"=refnum<k21> "IO Socket\\SI 1 Deserializer GPIO 5 Output Enable") -> ()  [unwired: 1 out]
              n152 = xnode "FPGA I/O Node"("I/O Item"=w343, "FPGA I/O In"=refnum<k21> "IO Socket\\SI 1 Deserializer GPIO 6 Output Enable") -> ()  [unwired: 1 out]
            }
            frame "SI 2 Deserializer" {
              n153 = xnode "FPGA I/O Node"("I/O Item"=w363, "FPGA I/O In"=refnum<k21> "IO Socket\\SI 2 Deserializer GPIO 0 Output Enable") -> ()  [unwired: 1 out]
              n154 = xnode "FPGA I/O Node"("I/O Item"=w362, "FPGA I/O In"=refnum<k21> "IO Socket\\SI 2 Deserializer GPIO 1 Output Enable") -> ()  [unwired: 1 out]
              n155 = xnode "FPGA I/O Node"("I/O Item"=w361, "FPGA I/O In"=refnum<k21> "IO Socket\\SI 2 Deserializer GPIO 2 Output Enable") -> ()  [unwired: 1 out]
              n156 = xnode "FPGA I/O Node"("I/O Item"=w360, "FPGA I/O In"=refnum<k21> "IO Socket\\SI 2 Deserializer GPIO 3 Output Enable") -> ()  [unwired: 1 out]
              n157 = xnode "FPGA I/O Node"("I/O Item"=w359, "FPGA I/O In"=refnum<k21> "IO Socket\\SI 2 Deserializer GPIO 4 Output Enable") -> ()  [unwired: 1 out]
              n158 = xnode "FPGA I/O Node"("I/O Item"=w358, "FPGA I/O In"=refnum<k21> "IO Socket\\SI 2 Deserializer GPIO 5 Output Enable") -> ()  [unwired: 1 out]
              n159 = xnode "FPGA I/O Node"("I/O Item"=w357, "FPGA I/O In"=refnum<k21> "IO Socket\\SI 2 Deserializer GPIO 6 Output Enable") -> ()  [unwired: 1 out]
            }
            frame "SI 3 Deserializer" {
              n160 = xnode "FPGA I/O Node"("I/O Item"=w377, "FPGA I/O In"=refnum<k21> "IO Socket\\SI 3 Deserializer GPIO 0 Output Enable") -> ()  [unwired: 1 out]
              n161 = xnode "FPGA I/O Node"("I/O Item"=w376, "FPGA I/O In"=refnum<k21> "IO Socket\\SI 3 Deserializer GPIO 1 Output Enable") -> ()  [unwired: 1 out]
              n162 = xnode "FPGA I/O Node"("I/O Item"=w375, "FPGA I/O In"=refnum<k21> "IO Socket\\SI 3 Deserializer GPIO 2 Output Enable") -> ()  [unwired: 1 out]
              n163 = xnode "FPGA I/O Node"("I/O Item"=w374, "FPGA I/O In"=refnum<k21> "IO Socket\\SI 3 Deserializer GPIO 3 Output Enable") -> ()  [unwired: 1 out]
              n164 = xnode "FPGA I/O Node"("I/O Item"=w373, "FPGA I/O In"=refnum<k21> "IO Socket\\SI 3 Deserializer GPIO 4 Output Enable") -> ()  [unwired: 1 out]
              n165 = xnode "FPGA I/O Node"("I/O Item"=w372, "FPGA I/O In"=refnum<k21> "IO Socket\\SI 3 Deserializer GPIO 5 Output Enable") -> ()  [unwired: 1 out]
              n166 = xnode "FPGA I/O Node"("I/O Item"=w371, "FPGA I/O In"=refnum<k21> "IO Socket\\SI 3 Deserializer GPIO 6 Output Enable") -> ()  [unwired: 1 out]
            }
            frame "SO 0 Serializer" {
              n167 = xnode "FPGA I/O Node"("I/O Item"=w388, "FPGA I/O In"=refnum<k21> "IO Socket\\SO 0 Serializer GPIO 0 Output Enable") -> ()  [unwired: 1 out]
              n168 = xnode "FPGA I/O Node"("I/O Item"=w387, "FPGA I/O In"=refnum<k21> "IO Socket\\SO 0 Serializer GPIO 1 Output Enable") -> ()  [unwired: 1 out]
              n169 = xnode "FPGA I/O Node"("I/O Item"=w386, "FPGA I/O In"=refnum<k21> "IO Socket\\SO 0 Serializer GPIO 2 Output Enable") -> ()  [unwired: 1 out]
              n170 = xnode "FPGA I/O Node"("I/O Item"=w385, "FPGA I/O In"=refnum<k21> "IO Socket\\SO 0 Serializer GPIO 3 Output Enable") -> ()  [unwired: 1 out]
            }
            frame "SO 1 Serializer" {
              n171 = xnode "FPGA I/O Node"("I/O Item"=w396, "FPGA I/O In"=refnum<k21> "IO Socket\\SO 1 Serializer GPIO 0 Output Enable") -> ()  [unwired: 1 out]
              n172 = xnode "FPGA I/O Node"("I/O Item"=w395, "FPGA I/O In"=refnum<k21> "IO Socket\\SO 1 Serializer GPIO 1 Output Enable") -> ()  [unwired: 1 out]
              n173 = xnode "FPGA I/O Node"("I/O Item"=w394, "FPGA I/O In"=refnum<k21> "IO Socket\\SO 1 Serializer GPIO 2 Output Enable") -> ()  [unwired: 1 out]
              n174 = xnode "FPGA I/O Node"("I/O Item"=w393, "FPGA I/O In"=refnum<k21> "IO Socket\\SO 1 Serializer GPIO 3 Output Enable") -> ()  [unwired: 1 out]
            }
            frame "SO 2 Serializer" {
              n175 = xnode "FPGA I/O Node"("I/O Item"=w404, "FPGA I/O In"=refnum<k21> "IO Socket\\SO 2 Serializer GPIO 0 Output Enable") -> ()  [unwired: 1 out]
              n176 = xnode "FPGA I/O Node"("I/O Item"=w403, "FPGA I/O In"=refnum<k21> "IO Socket\\SO 2 Serializer GPIO 1 Output Enable") -> ()  [unwired: 1 out]
              n177 = xnode "FPGA I/O Node"("I/O Item"=w402, "FPGA I/O In"=refnum<k21> "IO Socket\\SO 2 Serializer GPIO 2 Output Enable") -> ()  [unwired: 1 out]
              n178 = xnode "FPGA I/O Node"("I/O Item"=w401, "FPGA I/O In"=refnum<k21> "IO Socket\\SO 2 Serializer GPIO 3 Output Enable") -> ()  [unwired: 1 out]
            }
            frame "SO 3 Serializer" {
              n179 = xnode "FPGA I/O Node"("I/O Item"=w412, "FPGA I/O In"=refnum<k21> "IO Socket\\SO 3 Serializer GPIO 0 Output Enable") -> ()  [unwired: 1 out]
              n180 = xnode "FPGA I/O Node"("I/O Item"=w411, "FPGA I/O In"=refnum<k21> "IO Socket\\SO 3 Serializer GPIO 1 Output Enable") -> ()  [unwired: 1 out]
              n181 = xnode "FPGA I/O Node"("I/O Item"=w410, "FPGA I/O In"=refnum<k21> "IO Socket\\SO 3 Serializer GPIO 2 Output Enable") -> ()  [unwired: 1 out]
              n182 = xnode "FPGA I/O Node"("I/O Item"=w409, "FPGA I/O In"=refnum<k21> "IO Socket\\SO 3 Serializer GPIO 3 Output Enable") -> ()  [unwired: 1 out]
            }
          }
          n183 = Not(x=w319) -> (.not. x?=w318:bool)
        }
        frame condition #4 {
          n184 = case shown="\"SI 0 Deserializer\"" w429 {
            tunnel: w428 -> [_ w443 w463 w483 w503 w514 w522 w530 w538]
            tunnel: w427 -> [_ w442 w462 w482 w502 w513 w521 w529 w537]
            tunnel: w426 -> [_ w441 w461 w481 w501 w512 w520 w528 w536]
            tunnel: w425 -> [_ w440 w460 w480 w500 w511 w519 w527 w535]
            tunnel: w424 -> [_ w439 w459 w479 w499 _ _ _ _]
            tunnel: w423 -> [_ w438 w458 w478 w498 _ _ _ _]
            tunnel: w422 -> [_ w437 w457 w477 w497 _ _ _ _]
            tunnel: [w430 _ _ _ _ _ _ _ _] -> w421
            tunnel: w419 -> [_ w433 w451 w473 w493 _ _ _ _]
            tunnel: w418 -> [_ w432 w452 w472 w492 _ _ _ _]
            tunnel: w417 -> [_ w431 w453 w471 w491 _ _ _ _]
            frame Default {
              w430 = TRUE  # serdes id invalid
            }
            frame "SI 0 Deserializer" {
              n185 = xnode "FPGA I/O Node"("I/O Item"=w443, "FPGA I/O In"=refnum<k21> "IO Socket\\SI 0 Deserializer GPIO 0 Output Enable") -> ()  [unwired: 1 out]
              n186 = xnode "FPGA I/O Node"("I/O Item"=w442, "FPGA I/O In"=refnum<k21> "IO Socket\\SI 0 Deserializer GPIO 1 Output Enable") -> ()  [unwired: 1 out]
              n187 = xnode "FPGA I/O Node"("I/O Item"=w441, "FPGA I/O In"=refnum<k21> "IO Socket\\SI 0 Deserializer GPIO 2 Output Enable") -> ()  [unwired: 1 out]
              n188 = xnode "FPGA I/O Node"("I/O Item"=w440, "FPGA I/O In"=refnum<k21> "IO Socket\\SI 0 Deserializer GPIO 3 Output Enable") -> ()  [unwired: 1 out]
              n189 = xnode "FPGA I/O Node"("I/O Item"=w439, "FPGA I/O In"=refnum<k21> "IO Socket\\SI 0 Deserializer GPIO 4 Output Enable") -> ()  [unwired: 1 out]
              n190 = xnode "FPGA I/O Node"("I/O Item"=w438, "FPGA I/O In"=refnum<k21> "IO Socket\\SI 0 Deserializer GPIO 5 Output Enable") -> ()  [unwired: 1 out]
              n191 = xnode "FPGA I/O Node"("I/O Item"=w437, "FPGA I/O In"=refnum<k21> "IO Socket\\SI 0 Deserializer GPIO 6 Output Enable") -> ()  [unwired: 1 out]
              n192 = xnode "FPGA I/O Node"("I/O Item"=w433, "FPGA I/O In"=refnum<k21> "IO Socket\\SI 0 Deserializer GPIO 7 Output Enable") -> ()  [unwired: 1 out]
              n193 = xnode "FPGA I/O Node"("I/O Item"=w432, "FPGA I/O In"=refnum<k21> "IO Socket\\SI 0 Deserializer GPIO 9 Output Enable") -> ()  [unwired: 1 out]
              n194 = xnode "FPGA I/O Node"("I/O Item"=w431, "FPGA I/O In"=refnum<k21> "IO Socket\\SI 0 Deserializer GPIO 10 Output Enable") -> ()  [unwired: 1 out]
            }
            frame "SI 1 Deserializer" {
              n195 = xnode "FPGA I/O Node"("I/O Item"=w463, "FPGA I/O In"=refnum<k21> "IO Socket\\SI 1 Deserializer GPIO 0 Output Enable") -> ()  [unwired: 1 out]
              n196 = xnode "FPGA I/O Node"("I/O Item"=w462, "FPGA I/O In"=refnum<k21> "IO Socket\\SI 1 Deserializer GPIO 1 Output Enable") -> ()  [unwired: 1 out]
              n197 = xnode "FPGA I/O Node"("I/O Item"=w461, "FPGA I/O In"=refnum<k21> "IO Socket\\SI 1 Deserializer GPIO 2 Output Enable") -> ()  [unwired: 1 out]
              n198 = xnode "FPGA I/O Node"("I/O Item"=w460, "FPGA I/O In"=refnum<k21> "IO Socket\\SI 1 Deserializer GPIO 3 Output Enable") -> ()  [unwired: 1 out]
              n199 = xnode "FPGA I/O Node"("I/O Item"=w459, "FPGA I/O In"=refnum<k21> "IO Socket\\SI 1 Deserializer GPIO 4 Output Enable") -> ()  [unwired: 1 out]
              n200 = xnode "FPGA I/O Node"("I/O Item"=w458, "FPGA I/O In"=refnum<k21> "IO Socket\\SI 1 Deserializer GPIO 5 Output Enable") -> ()  [unwired: 1 out]
              n201 = xnode "FPGA I/O Node"("I/O Item"=w457, "FPGA I/O In"=refnum<k21> "IO Socket\\SI 1 Deserializer GPIO 6 Output Enable") -> ()  [unwired: 1 out]
              n202 = xnode "FPGA I/O Node"("I/O Item"=w451, "FPGA I/O In"=refnum<k21> "IO Socket\\SI 1 Deserializer GPIO 7 Output Enable") -> ()  [unwired: 1 out]
              n203 = xnode "FPGA I/O Node"("I/O Item"=w452, "FPGA I/O In"=refnum<k21> "IO Socket\\SI 1 Deserializer GPIO 9 Output Enable") -> ()  [unwired: 1 out]
              n204 = xnode "FPGA I/O Node"("I/O Item"=w453, "FPGA I/O In"=refnum<k21> "IO Socket\\SI 1 Deserializer GPIO 10 Output Enable") -> ()  [unwired: 1 out]
            }
            frame "SI 2 Deserializer" {
              n205 = xnode "FPGA I/O Node"("I/O Item"=w483, "FPGA I/O In"=refnum<k21> "IO Socket\\SI 2 Deserializer GPIO 0 Output Enable") -> ()  [unwired: 1 out]
              n206 = xnode "FPGA I/O Node"("I/O Item"=w482, "FPGA I/O In"=refnum<k21> "IO Socket\\SI 2 Deserializer GPIO 1 Output Enable") -> ()  [unwired: 1 out]
              n207 = xnode "FPGA I/O Node"("I/O Item"=w481, "FPGA I/O In"=refnum<k21> "IO Socket\\SI 2 Deserializer GPIO 2 Output Enable") -> ()  [unwired: 1 out]
              n208 = xnode "FPGA I/O Node"("I/O Item"=w480, "FPGA I/O In"=refnum<k21> "IO Socket\\SI 2 Deserializer GPIO 3 Output Enable") -> ()  [unwired: 1 out]
              n209 = xnode "FPGA I/O Node"("I/O Item"=w479, "FPGA I/O In"=refnum<k21> "IO Socket\\SI 2 Deserializer GPIO 4 Output Enable") -> ()  [unwired: 1 out]
              n210 = xnode "FPGA I/O Node"("I/O Item"=w478, "FPGA I/O In"=refnum<k21> "IO Socket\\SI 2 Deserializer GPIO 5 Output Enable") -> ()  [unwired: 1 out]
              n211 = xnode "FPGA I/O Node"("I/O Item"=w477, "FPGA I/O In"=refnum<k21> "IO Socket\\SI 2 Deserializer GPIO 6 Output Enable") -> ()  [unwired: 1 out]
              n212 = xnode "FPGA I/O Node"("I/O Item"=w473, "FPGA I/O In"=refnum<k21> "IO Socket\\SI 2 Deserializer GPIO 7 Output Enable") -> ()  [unwired: 1 out]
              n213 = xnode "FPGA I/O Node"("I/O Item"=w472, "FPGA I/O In"=refnum<k21> "IO Socket\\SI 2 Deserializer GPIO 9 Output Enable") -> ()  [unwired: 1 out]
              n214 = xnode "FPGA I/O Node"("I/O Item"=w471, "FPGA I/O In"=refnum<k21> "IO Socket\\SI 2 Deserializer GPIO 10 Output Enable") -> ()  [unwired: 1 out]
            }
            frame "SI 3 Deserializer" {
              n215 = xnode "FPGA I/O Node"("I/O Item"=w503, "FPGA I/O In"=refnum<k21> "IO Socket\\SI 3 Deserializer GPIO 0 Output Enable") -> ()  [unwired: 1 out]
              n216 = xnode "FPGA I/O Node"("I/O Item"=w502, "FPGA I/O In"=refnum<k21> "IO Socket\\SI 3 Deserializer GPIO 1 Output Enable") -> ()  [unwired: 1 out]
              n217 = xnode "FPGA I/O Node"("I/O Item"=w501, "FPGA I/O In"=refnum<k21> "IO Socket\\SI 3 Deserializer GPIO 2 Output Enable") -> ()  [unwired: 1 out]
              n218 = xnode "FPGA I/O Node"("I/O Item"=w500, "FPGA I/O In"=refnum<k21> "IO Socket\\SI 3 Deserializer GPIO 3 Output Enable") -> ()  [unwired: 1 out]
              n219 = xnode "FPGA I/O Node"("I/O Item"=w499, "FPGA I/O In"=refnum<k21> "IO Socket\\SI 3 Deserializer GPIO 4 Output Enable") -> ()  [unwired: 1 out]
              n220 = xnode "FPGA I/O Node"("I/O Item"=w498, "FPGA I/O In"=refnum<k21> "IO Socket\\SI 3 Deserializer GPIO 5 Output Enable") -> ()  [unwired: 1 out]
              n221 = xnode "FPGA I/O Node"("I/O Item"=w497, "FPGA I/O In"=refnum<k21> "IO Socket\\SI 3 Deserializer GPIO 6 Output Enable") -> ()  [unwired: 1 out]
              n222 = xnode "FPGA I/O Node"("I/O Item"=w493, "FPGA I/O In"=refnum<k21> "IO Socket\\SI 3 Deserializer GPIO 7 Output Enable") -> ()  [unwired: 1 out]
              n223 = xnode "FPGA I/O Node"("I/O Item"=w492, "FPGA I/O In"=refnum<k21> "IO Socket\\SI 3 Deserializer GPIO 9 Output Enable") -> ()  [unwired: 1 out]
              n224 = xnode "FPGA I/O Node"("I/O Item"=w491, "FPGA I/O In"=refnum<k21> "IO Socket\\SI 3 Deserializer GPIO 10 Output Enable") -> ()  [unwired: 1 out]
            }
            frame "SO 0 Serializer" {
              n225 = xnode "FPGA I/O Node"("I/O Item"=w514, "FPGA I/O In"=refnum<k21> "IO Socket\\SO 0 Serializer GPIO 0 Output Enable") -> ()  [unwired: 1 out]
              n226 = xnode "FPGA I/O Node"("I/O Item"=w513, "FPGA I/O In"=refnum<k21> "IO Socket\\SO 0 Serializer GPIO 1 Output Enable") -> ()  [unwired: 1 out]
              n227 = xnode "FPGA I/O Node"("I/O Item"=w512, "FPGA I/O In"=refnum<k21> "IO Socket\\SO 0 Serializer GPIO 2 Output Enable") -> ()  [unwired: 1 out]
              n228 = xnode "FPGA I/O Node"("I/O Item"=w511, "FPGA I/O In"=refnum<k21> "IO Socket\\SO 0 Serializer GPIO 3 Output Enable") -> ()  [unwired: 1 out]
            }
            frame "SO 1 Serializer" {
              n229 = xnode "FPGA I/O Node"("I/O Item"=w522, "FPGA I/O In"=refnum<k21> "IO Socket\\SO 1 Serializer GPIO 0 Output Enable") -> ()  [unwired: 1 out]
              n230 = xnode "FPGA I/O Node"("I/O Item"=w521, "FPGA I/O In"=refnum<k21> "IO Socket\\SO 1 Serializer GPIO 1 Output Enable") -> ()  [unwired: 1 out]
              n231 = xnode "FPGA I/O Node"("I/O Item"=w520, "FPGA I/O In"=refnum<k21> "IO Socket\\SO 1 Serializer GPIO 2 Output Enable") -> ()  [unwired: 1 out]
              n232 = xnode "FPGA I/O Node"("I/O Item"=w519, "FPGA I/O In"=refnum<k21> "IO Socket\\SO 1 Serializer GPIO 3 Output Enable") -> ()  [unwired: 1 out]
            }
            frame "SO 2 Serializer" {
              n233 = xnode "FPGA I/O Node"("I/O Item"=w530, "FPGA I/O In"=refnum<k21> "IO Socket\\SO 2 Serializer GPIO 0 Output Enable") -> ()  [unwired: 1 out]
              n234 = xnode "FPGA I/O Node"("I/O Item"=w529, "FPGA I/O In"=refnum<k21> "IO Socket\\SO 2 Serializer GPIO 1 Output Enable") -> ()  [unwired: 1 out]
              n235 = xnode "FPGA I/O Node"("I/O Item"=w528, "FPGA I/O In"=refnum<k21> "IO Socket\\SO 2 Serializer GPIO 2 Output Enable") -> ()  [unwired: 1 out]
              n236 = xnode "FPGA I/O Node"("I/O Item"=w527, "FPGA I/O In"=refnum<k21> "IO Socket\\SO 2 Serializer GPIO 3 Output Enable") -> ()  [unwired: 1 out]
            }
            frame "SO 3 Serializer" {
              n237 = xnode "FPGA I/O Node"("I/O Item"=w538, "FPGA I/O In"=refnum<k21> "IO Socket\\SO 3 Serializer GPIO 0 Output Enable") -> ()  [unwired: 1 out]
              n238 = xnode "FPGA I/O Node"("I/O Item"=w537, "FPGA I/O In"=refnum<k21> "IO Socket\\SO 3 Serializer GPIO 1 Output Enable") -> ()  [unwired: 1 out]
              n239 = xnode "FPGA I/O Node"("I/O Item"=w536, "FPGA I/O In"=refnum<k21> "IO Socket\\SO 3 Serializer GPIO 2 Output Enable") -> ()  [unwired: 1 out]
              n240 = xnode "FPGA I/O Node"("I/O Item"=w535, "FPGA I/O In"=refnum<k21> "IO Socket\\SO 3 Serializer GPIO 3 Output Enable") -> ()  [unwired: 1 out]
            }
          }
          n241 = Not(x=w421) -> (.not. x?=w420:bool)
        }
        frame condition #5 {
          n242 = case shown="\"SI 4 SI 5 Deserializer\"" w556 {
            tunnel: w555 -> [_ w570 w588 w606 w624]
            tunnel: w554 -> [_ w569 w587 w605 w623]
            tunnel: w553 -> [_ _ _ _ _]
            tunnel: w552 -> [_ _ _ _ _]
            tunnel: w551 -> [_ w568 w586 w604 w622]
            tunnel: w550 -> [_ w567 w585 w603 w621]
            tunnel: w549 -> [_ w566 w584 w602 w620]
            tunnel: [w557 _ _ _ _] -> w548
            tunnel: w546 -> [_ w564 w582 w600 w618]
            tunnel: w545 -> [_ w560 w578 w596 w614]
            tunnel: w544 -> [_ w559 w577 w595 w613]
            tunnel: w543 -> [_ w558 w576 w594 w612]
            frame Default {
              w557 = TRUE  # serdes id invalid
            }
            frame "SI 0 SI 1 Deserializer" {
              n243 = xnode "FPGA I/O Node"("I/O Item"=w570, "FPGA I/O In"=refnum<k21> "IO Socket\\SI 0 SI 1 Deserializer MFP 0 Output Enable") -> ()  [unwired: 1 out]
              n244 = xnode "FPGA I/O Node"("I/O Item"=w569, "FPGA I/O In"=refnum<k21> "IO Socket\\SI 0 SI 1 Deserializer MFP 1 Output Enable") -> ()  [unwired: 1 out]
              n245 = xnode "FPGA I/O Node"("I/O Item"=w568, "FPGA I/O In"=refnum<k21> "IO Socket\\SI 0 SI 1 Deserializer MFP 4 Output Enable") -> ()  [unwired: 1 out]
              n246 = xnode "FPGA I/O Node"("I/O Item"=w567, "FPGA I/O In"=refnum<k21> "IO Socket\\SI 0 SI 1 Deserializer MFP 5 Output Enable") -> ()  [unwired: 1 out]
              n247 = xnode "FPGA I/O Node"("I/O Item"=w566, "FPGA I/O In"=refnum<k21> "IO Socket\\SI 0 SI 1 Deserializer MFP 6 Output Enable") -> ()  [unwired: 1 out]
              n248 = xnode "FPGA I/O Node"("I/O Item"=w564, "FPGA I/O In"=refnum<k21> "IO Socket\\SI 0 SI 1 Deserializer MFP 7 Output Enable") -> ()  [unwired: 1 out]
              n249 = xnode "FPGA I/O Node"("I/O Item"=w560, "FPGA I/O In"=refnum<k21> "IO Socket\\SI 0 SI 1 Deserializer MFP 8 Output Enable") -> ()  [unwired: 1 out]
              n250 = xnode "FPGA I/O Node"("I/O Item"=w559, "FPGA I/O In"=refnum<k21> "IO Socket\\SI 0 SI 1 Deserializer MFP 9 Output Enable") -> ()  [unwired: 1 out]
              n251 = xnode "FPGA I/O Node"("I/O Item"=w558, "FPGA I/O In"=refnum<k21> "IO Socket\\SI 0 SI 1 Deserializer MFP 10 Output Enable") -> ()  [unwired: 1 out]
            }
            frame "SI 2 SI 3 Deserializer" {
              n252 = xnode "FPGA I/O Node"("I/O Item"=w588, "FPGA I/O In"=refnum<k21> "IO Socket\\SI 2 SI 3 Deserializer MFP 0 Output Enable") -> ()  [unwired: 1 out]
              n253 = xnode "FPGA I/O Node"("I/O Item"=w587, "FPGA I/O In"=refnum<k21> "IO Socket\\SI 2 SI 3 Deserializer MFP 1 Output Enable") -> ()  [unwired: 1 out]
              n254 = xnode "FPGA I/O Node"("I/O Item"=w586, "FPGA I/O In"=refnum<k21> "IO Socket\\SI 2 SI 3 Deserializer MFP 4 Output Enable") -> ()  [unwired: 1 out]
              n255 = xnode "FPGA I/O Node"("I/O Item"=w585, "FPGA I/O In"=refnum<k21> "IO Socket\\SI 2 SI 3 Deserializer MFP 5 Output Enable") -> ()  [unwired: 1 out]
              n256 = xnode "FPGA I/O Node"("I/O Item"=w584, "FPGA I/O In"=refnum<k21> "IO Socket\\SI 2 SI 3 Deserializer MFP 6 Output Enable") -> ()  [unwired: 1 out]
              n257 = xnode "FPGA I/O Node"("I/O Item"=w582, "FPGA I/O In"=refnum<k21> "IO Socket\\SI 2 SI 3 Deserializer MFP 7 Output Enable") -> ()  [unwired: 1 out]
              n258 = xnode "FPGA I/O Node"("I/O Item"=w578, "FPGA I/O In"=refnum<k21> "IO Socket\\SI 2 SI 3 Deserializer MFP 8 Output Enable") -> ()  [unwired: 1 out]
              n259 = xnode "FPGA I/O Node"("I/O Item"=w577, "FPGA I/O In"=refnum<k21> "IO Socket\\SI 2 SI 3 Deserializer MFP 9 Output Enable") -> ()  [unwired: 1 out]
              n260 = xnode "FPGA I/O Node"("I/O Item"=w576, "FPGA I/O In"=refnum<k21> "IO Socket\\SI 2 SI 3 Deserializer MFP 10 Output Enable") -> ()  [unwired: 1 out]
            }
            frame "SI 4 SI 5 Deserializer" {
              n261 = xnode "FPGA I/O Node"("I/O Item"=w606, "FPGA I/O In"=refnum<k21> "IO Socket\\SI 4 SI 5 Deserializer MFP 0 Output Enable") -> ()  [unwired: 1 out]
              n262 = xnode "FPGA I/O Node"("I/O Item"=w605, "FPGA I/O In"=refnum<k21> "IO Socket\\SI 4 SI 5 Deserializer MFP 1 Output Enable") -> ()  [unwired: 1 out]
              n263 = xnode "FPGA I/O Node"("I/O Item"=w604, "FPGA I/O In"=refnum<k21> "IO Socket\\SI 4 SI 5 Deserializer MFP 4 Output Enable") -> ()  [unwired: 1 out]
              n264 = xnode "FPGA I/O Node"("I/O Item"=w603, "FPGA I/O In"=refnum<k21> "IO Socket\\SI 4 SI 5 Deserializer MFP 5 Output Enable") -> ()  [unwired: 1 out]
              n265 = xnode "FPGA I/O Node"("I/O Item"=w602, "FPGA I/O In"=refnum<k21> "IO Socket\\SI 4 SI 5 Deserializer MFP 6 Output Enable") -> ()  [unwired: 1 out]
              n266 = xnode "FPGA I/O Node"("I/O Item"=w600, "FPGA I/O In"=refnum<k21> "IO Socket\\SI 4 SI 5 Deserializer MFP 7 Output Enable") -> ()  [unwired: 1 out]
              n267 = xnode "FPGA I/O Node"("I/O Item"=w596, "FPGA I/O In"=refnum<k21> "IO Socket\\SI 4 SI 5 Deserializer MFP 8 Output Enable") -> ()  [unwired: 1 out]
              n268 = xnode "FPGA I/O Node"("I/O Item"=w595, "FPGA I/O In"=refnum<k21> "IO Socket\\SI 4 SI 5 Deserializer MFP 9 Output Enable") -> ()  [unwired: 1 out]
              n269 = xnode "FPGA I/O Node"("I/O Item"=w594, "FPGA I/O In"=refnum<k21> "IO Socket\\SI 4 SI 5 Deserializer MFP 10 Output Enable") -> ()  [unwired: 1 out]
            }
            frame "SI 6 SI 7 Deserializer" {
              n270 = xnode "FPGA I/O Node"("I/O Item"=w624, "FPGA I/O In"=refnum<k21> "IO Socket\\SI 6 SI 7 Deserializer MFP 0 Output Enable") -> ()  [unwired: 1 out]
              n271 = xnode "FPGA I/O Node"("I/O Item"=w623, "FPGA I/O In"=refnum<k21> "IO Socket\\SI 6 SI 7 Deserializer MFP 1 Output Enable") -> ()  [unwired: 1 out]
              n272 = xnode "FPGA I/O Node"("I/O Item"=w622, "FPGA I/O In"=refnum<k21> "IO Socket\\SI 6 SI 7 Deserializer MFP 4 Output Enable") -> ()  [unwired: 1 out]
              n273 = xnode "FPGA I/O Node"("I/O Item"=w621, "FPGA I/O In"=refnum<k21> "IO Socket\\SI 6 SI 7 Deserializer MFP 5 Output Enable") -> ()  [unwired: 1 out]
              n274 = xnode "FPGA I/O Node"("I/O Item"=w620, "FPGA I/O In"=refnum<k21> "IO Socket\\SI 6 SI 7 Deserializer MFP 6 Output Enable") -> ()  [unwired: 1 out]
              n275 = xnode "FPGA I/O Node"("I/O Item"=w618, "FPGA I/O In"=refnum<k21> "IO Socket\\SI 6 SI 7 Deserializer MFP 7 Output Enable") -> ()  [unwired: 1 out]
              n276 = xnode "FPGA I/O Node"("I/O Item"=w614, "FPGA I/O In"=refnum<k21> "IO Socket\\SI 6 SI 7 Deserializer MFP 8 Output Enable") -> ()  [unwired: 1 out]
              n277 = xnode "FPGA I/O Node"("I/O Item"=w613, "FPGA I/O In"=refnum<k21> "IO Socket\\SI 6 SI 7 Deserializer MFP 9 Output Enable") -> ()  [unwired: 1 out]
              n278 = xnode "FPGA I/O Node"("I/O Item"=w612, "FPGA I/O In"=refnum<k21> "IO Socket\\SI 6 SI 7 Deserializer MFP 10 Output Enable") -> ()  [unwired: 1 out]
            }
          }
          n279 = Not(x=w548) -> (.not. x?=w547:bool)
        }
        frame condition #6 {
          n280 = case shown="\"SI 2 SI 3 Deserializer\"" w643 {
            tunnel: w642 -> [_ w657 w675]
            tunnel: w641 -> [_ w656 w674]
            tunnel: w640 -> [_ _ _]
            tunnel: w639 -> [_ _ _]
            tunnel: w638 -> [_ w655 w673]
            tunnel: w637 -> [_ w654 w672]
            tunnel: w636 -> [_ w653 w671]
            tunnel: [w644 _ _] -> w635
            tunnel: w633 -> [_ w651 w669]
            tunnel: w632 -> [_ w647 w665]
            tunnel: w631 -> [_ w646 w664]
            tunnel: w630 -> [_ w645 w663]
            frame Default {
              w644 = TRUE  # serdes id invalid
            }
            frame "SI 0 SI 1 Deserializer" {
              n281 = xnode "FPGA I/O Node"("I/O Item"=w657, "FPGA I/O In"=refnum<k21> "IO Socket\\SI 0 SI 1 Deserializer MFP 0 Output Enable") -> ()  [unwired: 1 out]
              n282 = xnode "FPGA I/O Node"("I/O Item"=w656, "FPGA I/O In"=refnum<k21> "IO Socket\\SI 0 SI 1 Deserializer MFP 1 Output Enable") -> ()  [unwired: 1 out]
              n283 = xnode "FPGA I/O Node"("I/O Item"=w655, "FPGA I/O In"=refnum<k21> "IO Socket\\SI 0 SI 1 Deserializer MFP 4 Output Enable") -> ()  [unwired: 1 out]
              n284 = xnode "FPGA I/O Node"("I/O Item"=w654, "FPGA I/O In"=refnum<k21> "IO Socket\\SI 0 SI 1 Deserializer MFP 5 Output Enable") -> ()  [unwired: 1 out]
              n285 = xnode "FPGA I/O Node"("I/O Item"=w653, "FPGA I/O In"=refnum<k21> "IO Socket\\SI 0 SI 1 Deserializer MFP 6 Output Enable") -> ()  [unwired: 1 out]
              n286 = xnode "FPGA I/O Node"("I/O Item"=w651, "FPGA I/O In"=refnum<k21> "IO Socket\\SI 0 SI 1 Deserializer MFP 7 Output Enable") -> ()  [unwired: 1 out]
              n287 = xnode "FPGA I/O Node"("I/O Item"=w647, "FPGA I/O In"=refnum<k21> "IO Socket\\SI 0 SI 1 Deserializer MFP 8 Output Enable") -> ()  [unwired: 1 out]
              n288 = xnode "FPGA I/O Node"("I/O Item"=w646, "FPGA I/O In"=refnum<k21> "IO Socket\\SI 0 SI 1 Deserializer MFP 9 Output Enable") -> ()  [unwired: 1 out]
              n289 = xnode "FPGA I/O Node"("I/O Item"=w645, "FPGA I/O In"=refnum<k21> "IO Socket\\SI 0 SI 1 Deserializer MFP 10 Output Enable") -> ()  [unwired: 1 out]
            }
            frame "SI 2 SI 3 Deserializer" {
              n290 = xnode "FPGA I/O Node"("I/O Item"=w675, "FPGA I/O In"=refnum<k21> "IO Socket\\SI 2 SI 3 Deserializer MFP 0 Output Enable") -> ()  [unwired: 1 out]
              n291 = xnode "FPGA I/O Node"("I/O Item"=w674, "FPGA I/O In"=refnum<k21> "IO Socket\\SI 2 SI 3 Deserializer MFP 1 Output Enable") -> ()  [unwired: 1 out]
              n292 = xnode "FPGA I/O Node"("I/O Item"=w673, "FPGA I/O In"=refnum<k21> "IO Socket\\SI 2 SI 3 Deserializer MFP 4 Output Enable") -> ()  [unwired: 1 out]
              n293 = xnode "FPGA I/O Node"("I/O Item"=w672, "FPGA I/O In"=refnum<k21> "IO Socket\\SI 2 SI 3 Deserializer MFP 5 Output Enable") -> ()  [unwired: 1 out]
              n294 = xnode "FPGA I/O Node"("I/O Item"=w671, "FPGA I/O In"=refnum<k21> "IO Socket\\SI 2 SI 3 Deserializer MFP 6 Output Enable") -> ()  [unwired: 1 out]
              n295 = xnode "FPGA I/O Node"("I/O Item"=w669, "FPGA I/O In"=refnum<k21> "IO Socket\\SI 2 SI 3 Deserializer MFP 7 Output Enable") -> ()  [unwired: 1 out]
              n296 = xnode "FPGA I/O Node"("I/O Item"=w665, "FPGA I/O In"=refnum<k21> "IO Socket\\SI 2 SI 3 Deserializer MFP 8 Output Enable") -> ()  [unwired: 1 out]
              n297 = xnode "FPGA I/O Node"("I/O Item"=w664, "FPGA I/O In"=refnum<k21> "IO Socket\\SI 2 SI 3 Deserializer MFP 9 Output Enable") -> ()  [unwired: 1 out]
              n298 = xnode "FPGA I/O Node"("I/O Item"=w663, "FPGA I/O In"=refnum<k21> "IO Socket\\SI 2 SI 3 Deserializer MFP 10 Output Enable") -> ()  [unwired: 1 out]
            }
          }
          n299 = Not(x=w635) -> (.not. x?=w634:bool)
        }
        frame condition #7 {
          n300 = case shown="\"SO 4 Serializer\"" w689 {
            tunnel: w688 -> [_ w700 w712 w724 w736 w748 w760 w772 w784]
            tunnel: w687 -> [_ w699 w711 w723 w735 w747 w759 w771 w783]
            tunnel: w686 -> [_ w695 w707 w719 w731 w743 w755 w767 w779]
            tunnel: w685 -> [_ w694 w706 w718 w730 w742 w754 w766 w778]
            tunnel: [w690 _ _ _ _ _ _ _ _] -> w684
            tunnel: w682 -> [_ w693 w705 w717 w729 w741 w753 w765 w777]
            tunnel: w681 -> [_ w691 w703 w715 w727 w739 w751 w763 w775]
            frame Default {
              w690 = TRUE  # serdes id invalid
            }
            frame "SO 0 Serializer" {
              n301 = xnode "FPGA I/O Node"("I/O Item"=w700, "FPGA I/O In"=refnum<k21> "IO Socket\\SO 0 Serializer MFP 0 Output Enable") -> ()  [unwired: 1 out]
              n302 = xnode "FPGA I/O Node"("I/O Item"=w699, "FPGA I/O In"=refnum<k21> "IO Socket\\SO 0 Serializer MFP 3 Output Enable") -> ()  [unwired: 1 out]
              n303 = xnode "FPGA I/O Node"("I/O Item"=w695, "FPGA I/O In"=refnum<k21> "IO Socket\\SO 0 Serializer MFP 4 Output Enable") -> ()  [unwired: 1 out]
              n304 = xnode "FPGA I/O Node"("I/O Item"=w694, "FPGA I/O In"=refnum<k21> "IO Socket\\SO 0 Serializer MFP 6 Output Enable") -> ()  [unwired: 1 out]
              n305 = xnode "FPGA I/O Node"("I/O Item"=w693, "FPGA I/O In"=refnum<k21> "IO Socket\\SO 0 Serializer MFP 7 Output Enable") -> ()  [unwired: 1 out]
              n306 = xnode "FPGA I/O Node"("I/O Item"=w691, "FPGA I/O In"=refnum<k21> "IO Socket\\SO 0 Serializer MFP 8 Output Enable") -> ()  [unwired: 1 out]
            }
            frame "SO 1 Serializer" {
              n307 = xnode "FPGA I/O Node"("I/O Item"=w712, "FPGA I/O In"=refnum<k21> "IO Socket\\SO 1 Serializer MFP 0 Output Enable") -> ()  [unwired: 1 out]
              n308 = xnode "FPGA I/O Node"("I/O Item"=w711, "FPGA I/O In"=refnum<k21> "IO Socket\\SO 1 Serializer MFP 3 Output Enable") -> ()  [unwired: 1 out]
              n309 = xnode "FPGA I/O Node"("I/O Item"=w707, "FPGA I/O In"=refnum<k21> "IO Socket\\SO 1 Serializer MFP 4 Output Enable") -> ()  [unwired: 1 out]
              n310 = xnode "FPGA I/O Node"("I/O Item"=w706, "FPGA I/O In"=refnum<k21> "IO Socket\\SO 1 Serializer MFP 6 Output Enable") -> ()  [unwired: 1 out]
              n311 = xnode "FPGA I/O Node"("I/O Item"=w705, "FPGA I/O In"=refnum<k21> "IO Socket\\SO 1 Serializer MFP 7 Output Enable") -> ()  [unwired: 1 out]
              n312 = xnode "FPGA I/O Node"("I/O Item"=w703, "FPGA I/O In"=refnum<k21> "IO Socket\\SO 1 Serializer MFP 8 Output Enable") -> ()  [unwired: 1 out]
            }
            frame "SO 2 Serializer" {
              n313 = xnode "FPGA I/O Node"("I/O Item"=w724, "FPGA I/O In"=refnum<k21> "IO Socket\\SO 2 Serializer MFP 0 Output Enable") -> ()  [unwired: 1 out]
              n314 = xnode "FPGA I/O Node"("I/O Item"=w723, "FPGA I/O In"=refnum<k21> "IO Socket\\SO 2 Serializer MFP 3 Output Enable") -> ()  [unwired: 1 out]
              n315 = xnode "FPGA I/O Node"("I/O Item"=w719, "FPGA I/O In"=refnum<k21> "IO Socket\\SO 2 Serializer MFP 4 Output Enable") -> ()  [unwired: 1 out]
              n316 = xnode "FPGA I/O Node"("I/O Item"=w718, "FPGA I/O In"=refnum<k21> "IO Socket\\SO 2 Serializer MFP 6 Output Enable") -> ()  [unwired: 1 out]
              n317 = xnode "FPGA I/O Node"("I/O Item"=w717, "FPGA I/O In"=refnum<k21> "IO Socket\\SO 2 Serializer MFP 7 Output Enable") -> ()  [unwired: 1 out]
              n318 = xnode "FPGA I/O Node"("I/O Item"=w715, "FPGA I/O In"=refnum<k21> "IO Socket\\SO 2 Serializer MFP 8 Output Enable") -> ()  [unwired: 1 out]
            }
            frame "SO 3 Serializer" {
              n319 = xnode "FPGA I/O Node"("I/O Item"=w736, "FPGA I/O In"=refnum<k21> "IO Socket\\SO 3 Serializer MFP 0 Output Enable") -> ()  [unwired: 1 out]
              n320 = xnode "FPGA I/O Node"("I/O Item"=w735, "FPGA I/O In"=refnum<k21> "IO Socket\\SO 3 Serializer MFP 3 Output Enable") -> ()  [unwired: 1 out]
              n321 = xnode "FPGA I/O Node"("I/O Item"=w731, "FPGA I/O In"=refnum<k21> "IO Socket\\SO 3 Serializer MFP 4 Output Enable") -> ()  [unwired: 1 out]
              n322 = xnode "FPGA I/O Node"("I/O Item"=w730, "FPGA I/O In"=refnum<k21> "IO Socket\\SO 3 Serializer MFP 6 Output Enable") -> ()  [unwired: 1 out]
              n323 = xnode "FPGA I/O Node"("I/O Item"=w729, "FPGA I/O In"=refnum<k21> "IO Socket\\SO 3 Serializer MFP 7 Output Enable") -> ()  [unwired: 1 out]
              n324 = xnode "FPGA I/O Node"("I/O Item"=w727, "FPGA I/O In"=refnum<k21> "IO Socket\\SO 3 Serializer MFP 8 Output Enable") -> ()  [unwired: 1 out]
            }
            frame "SO 4 Serializer" {
              n325 = xnode "FPGA I/O Node"("I/O Item"=w748, "FPGA I/O In"=refnum<k21> "IO Socket\\SO 4 Serializer MFP 0 Output Enable") -> ()  [unwired: 1 out]
              n326 = xnode "FPGA I/O Node"("I/O Item"=w747, "FPGA I/O In"=refnum<k21> "IO Socket\\SO 4 Serializer MFP 3 Output Enable") -> ()  [unwired: 1 out]
              n327 = xnode "FPGA I/O Node"("I/O Item"=w743, "FPGA I/O In"=refnum<k21> "IO Socket\\SO 4 Serializer MFP 4 Output Enable") -> ()  [unwired: 1 out]
              n328 = xnode "FPGA I/O Node"("I/O Item"=w742, "FPGA I/O In"=refnum<k21> "IO Socket\\SO 4 Serializer MFP 6 Output Enable") -> ()  [unwired: 1 out]
              n329 = xnode "FPGA I/O Node"("I/O Item"=w741, "FPGA I/O In"=refnum<k21> "IO Socket\\SO 4 Serializer MFP 7 Output Enable") -> ()  [unwired: 1 out]
              n330 = xnode "FPGA I/O Node"("I/O Item"=w739, "FPGA I/O In"=refnum<k21> "IO Socket\\SO 4 Serializer MFP 8 Output Enable") -> ()  [unwired: 1 out]
            }
            frame "SO 5 Serializer" {
              n331 = xnode "FPGA I/O Node"("I/O Item"=w760, "FPGA I/O In"=refnum<k21> "IO Socket\\SO 5 Serializer MFP 0 Output Enable") -> ()  [unwired: 1 out]
              n332 = xnode "FPGA I/O Node"("I/O Item"=w759, "FPGA I/O In"=refnum<k21> "IO Socket\\SO 5 Serializer MFP 3 Output Enable") -> ()  [unwired: 1 out]
              n333 = xnode "FPGA I/O Node"("I/O Item"=w755, "FPGA I/O In"=refnum<k21> "IO Socket\\SO 5 Serializer MFP 4 Output Enable") -> ()  [unwired: 1 out]
              n334 = xnode "FPGA I/O Node"("I/O Item"=w754, "FPGA I/O In"=refnum<k21> "IO Socket\\SO 5 Serializer MFP 6 Output Enable") -> ()  [unwired: 1 out]
              n335 = xnode "FPGA I/O Node"("I/O Item"=w753, "FPGA I/O In"=refnum<k21> "IO Socket\\SO 5 Serializer MFP 7 Output Enable") -> ()  [unwired: 1 out]
              n336 = xnode "FPGA I/O Node"("I/O Item"=w751, "FPGA I/O In"=refnum<k21> "IO Socket\\SO 5 Serializer MFP 8 Output Enable") -> ()  [unwired: 1 out]
            }
            frame "SO 6 Serializer" {
              n337 = xnode "FPGA I/O Node"("I/O Item"=w772, "FPGA I/O In"=refnum<k21> "IO Socket\\SO 6 Serializer MFP 0 Output Enable") -> ()  [unwired: 1 out]
              n338 = xnode "FPGA I/O Node"("I/O Item"=w771, "FPGA I/O In"=refnum<k21> "IO Socket\\SO 6 Serializer MFP 3 Output Enable") -> ()  [unwired: 1 out]
              n339 = xnode "FPGA I/O Node"("I/O Item"=w767, "FPGA I/O In"=refnum<k21> "IO Socket\\SO 6 Serializer MFP 4 Output Enable") -> ()  [unwired: 1 out]
              n340 = xnode "FPGA I/O Node"("I/O Item"=w766, "FPGA I/O In"=refnum<k21> "IO Socket\\SO 6 Serializer MFP 6 Output Enable") -> ()  [unwired: 1 out]
              n341 = xnode "FPGA I/O Node"("I/O Item"=w765, "FPGA I/O In"=refnum<k21> "IO Socket\\SO 6 Serializer MFP 7 Output Enable") -> ()  [unwired: 1 out]
              n342 = xnode "FPGA I/O Node"("I/O Item"=w763, "FPGA I/O In"=refnum<k21> "IO Socket\\SO 6 Serializer MFP 8 Output Enable") -> ()  [unwired: 1 out]
            }
            frame "SO 7 Serializer" {
              n343 = xnode "FPGA I/O Node"("I/O Item"=w784, "FPGA I/O In"=refnum<k21> "IO Socket\\SO 7 Serializer MFP 0 Output Enable") -> ()  [unwired: 1 out]
              n344 = xnode "FPGA I/O Node"("I/O Item"=w783, "FPGA I/O In"=refnum<k21> "IO Socket\\SO 7 Serializer MFP 3 Output Enable") -> ()  [unwired: 1 out]
              n345 = xnode "FPGA I/O Node"("I/O Item"=w779, "FPGA I/O In"=refnum<k21> "IO Socket\\SO 7 Serializer MFP 4 Output Enable") -> ()  [unwired: 1 out]
              n346 = xnode "FPGA I/O Node"("I/O Item"=w778, "FPGA I/O In"=refnum<k21> "IO Socket\\SO 7 Serializer MFP 6 Output Enable") -> ()  [unwired: 1 out]
              n347 = xnode "FPGA I/O Node"("I/O Item"=w777, "FPGA I/O In"=refnum<k21> "IO Socket\\SO 7 Serializer MFP 7 Output Enable") -> ()  [unwired: 1 out]
              n348 = xnode "FPGA I/O Node"("I/O Item"=w775, "FPGA I/O In"=refnum<k21> "IO Socket\\SO 7 Serializer MFP 8 Output Enable") -> ()  [unwired: 1 out]
            }
          }
          n349 = Not(x=w684) -> (.not. x?=w683:bool)
        }
        frame condition #8 {
          n350 = case shown="\"SO 3 Serializer\"" w795 {
            tunnel: w794 -> [_ w806 w818 w830 w842]
            tunnel: w793 -> [_ w805 w817 w829 w841]
            tunnel: w792 -> [_ w801 w813 w825 w837]
            tunnel: w791 -> [_ w800 w812 w824 w836]
            tunnel: [w796 _ _ _ _] -> w790
            tunnel: w788 -> [_ w799 w811 w823 w835]
            tunnel: w787 -> [_ w797 w809 w821 w833]
            frame Default {
              w796 = TRUE  # serdes id invalid
            }
            frame "SO 0 Serializer" {
              n351 = xnode "FPGA I/O Node"("I/O Item"=w806, "FPGA I/O In"=refnum<k21> "IO Socket\\SO 0 Serializer MFP 0 Output Enable") -> ()  [unwired: 1 out]
              n352 = xnode "FPGA I/O Node"("I/O Item"=w805, "FPGA I/O In"=refnum<k21> "IO Socket\\SO 0 Serializer MFP 3 Output Enable") -> ()  [unwired: 1 out]
              n353 = xnode "FPGA I/O Node"("I/O Item"=w801, "FPGA I/O In"=refnum<k21> "IO Socket\\SO 0 Serializer MFP 4 Output Enable") -> ()  [unwired: 1 out]
              n354 = xnode "FPGA I/O Node"("I/O Item"=w800, "FPGA I/O In"=refnum<k21> "IO Socket\\SO 0 Serializer MFP 6 Output Enable") -> ()  [unwired: 1 out]
              n355 = xnode "FPGA I/O Node"("I/O Item"=w799, "FPGA I/O In"=refnum<k21> "IO Socket\\SO 0 Serializer MFP 7 Output Enable") -> ()  [unwired: 1 out]
              n356 = xnode "FPGA I/O Node"("I/O Item"=w797, "FPGA I/O In"=refnum<k21> "IO Socket\\SO 0 Serializer MFP 8 Output Enable") -> ()  [unwired: 1 out]
            }
            frame "SO 1 Serializer" {
              n357 = xnode "FPGA I/O Node"("I/O Item"=w818, "FPGA I/O In"=refnum<k21> "IO Socket\\SO 1 Serializer MFP 0 Output Enable") -> ()  [unwired: 1 out]
              n358 = xnode "FPGA I/O Node"("I/O Item"=w817, "FPGA I/O In"=refnum<k21> "IO Socket\\SO 1 Serializer MFP 3 Output Enable") -> ()  [unwired: 1 out]
              n359 = xnode "FPGA I/O Node"("I/O Item"=w813, "FPGA I/O In"=refnum<k21> "IO Socket\\SO 1 Serializer MFP 4 Output Enable") -> ()  [unwired: 1 out]
              n360 = xnode "FPGA I/O Node"("I/O Item"=w812, "FPGA I/O In"=refnum<k21> "IO Socket\\SO 1 Serializer MFP 6 Output Enable") -> ()  [unwired: 1 out]
              n361 = xnode "FPGA I/O Node"("I/O Item"=w811, "FPGA I/O In"=refnum<k21> "IO Socket\\SO 1 Serializer MFP 7 Output Enable") -> ()  [unwired: 1 out]
              n362 = xnode "FPGA I/O Node"("I/O Item"=w809, "FPGA I/O In"=refnum<k21> "IO Socket\\SO 1 Serializer MFP 8 Output Enable") -> ()  [unwired: 1 out]
            }
            frame "SO 2 Serializer" {
              n363 = xnode "FPGA I/O Node"("I/O Item"=w830, "FPGA I/O In"=refnum<k21> "IO Socket\\SO 2 Serializer MFP 0 Output Enable") -> ()  [unwired: 1 out]
              n364 = xnode "FPGA I/O Node"("I/O Item"=w829, "FPGA I/O In"=refnum<k21> "IO Socket\\SO 2 Serializer MFP 3 Output Enable") -> ()  [unwired: 1 out]
              n365 = xnode "FPGA I/O Node"("I/O Item"=w825, "FPGA I/O In"=refnum<k21> "IO Socket\\SO 2 Serializer MFP 4 Output Enable") -> ()  [unwired: 1 out]
              n366 = xnode "FPGA I/O Node"("I/O Item"=w824, "FPGA I/O In"=refnum<k21> "IO Socket\\SO 2 Serializer MFP 6 Output Enable") -> ()  [unwired: 1 out]
              n367 = xnode "FPGA I/O Node"("I/O Item"=w823, "FPGA I/O In"=refnum<k21> "IO Socket\\SO 2 Serializer MFP 7 Output Enable") -> ()  [unwired: 1 out]
              n368 = xnode "FPGA I/O Node"("I/O Item"=w821, "FPGA I/O In"=refnum<k21> "IO Socket\\SO 2 Serializer MFP 8 Output Enable") -> ()  [unwired: 1 out]
            }
            frame "SO 3 Serializer" {
              n369 = xnode "FPGA I/O Node"("I/O Item"=w842, "FPGA I/O In"=refnum<k21> "IO Socket\\SO 3 Serializer MFP 0 Output Enable") -> ()  [unwired: 1 out]
              n370 = xnode "FPGA I/O Node"("I/O Item"=w841, "FPGA I/O In"=refnum<k21> "IO Socket\\SO 3 Serializer MFP 3 Output Enable") -> ()  [unwired: 1 out]
              n371 = xnode "FPGA I/O Node"("I/O Item"=w837, "FPGA I/O In"=refnum<k21> "IO Socket\\SO 3 Serializer MFP 4 Output Enable") -> ()  [unwired: 1 out]
              n372 = xnode "FPGA I/O Node"("I/O Item"=w836, "FPGA I/O In"=refnum<k21> "IO Socket\\SO 3 Serializer MFP 6 Output Enable") -> ()  [unwired: 1 out]
              n373 = xnode "FPGA I/O Node"("I/O Item"=w835, "FPGA I/O In"=refnum<k21> "IO Socket\\SO 3 Serializer MFP 7 Output Enable") -> ()  [unwired: 1 out]
              n374 = xnode "FPGA I/O Node"("I/O Item"=w833, "FPGA I/O In"=refnum<k21> "IO Socket\\SO 3 Serializer MFP 8 Output Enable") -> ()  [unwired: 1 out]
            }
          }
          n375 = Not(x=w790) -> (.not. x?=w789:bool)
        }
        frame condition #9 {
          n376 = case shown="\"SI 3 Deserializer\"" w858 {
            tunnel: w857 -> [_ w872 w890 w908 w926 w941 w953 w965 w977]
            tunnel: w856 -> [_ w871 w889 w907 w925 _ _ _ _]
            tunnel: w855 -> [_ _ _ _ _ _ _ _ _]
            tunnel: w854 -> [_ _ _ _ _ w940 w952 w964 w976]
            tunnel: w853 -> [_ w870 w888 w906 w924 w936 w948 w960 w972]
            tunnel: w852 -> [_ w869 w887 w905 w923 _ _ _ _]
            tunnel: w851 -> [_ w868 w886 w904 w922 w935 w947 w959 w971]
            tunnel: [w859 _ _ _ _ _ _ _ _] -> w850
            tunnel: w848 -> [_ w860 w878 w896 w914 w934 w946 w958 w970]
            tunnel: w847 -> [_ w861 w879 w897 w915 w932 w944 w956 w968]
            tunnel: w846 -> [_ w862 w880 w898 w916 _ _ _ _]
            tunnel: w845 -> [_ w863 w881 w899 w917 _ _ _ _]
            frame Default {
              w859 = TRUE  # serdes id invalid
            }
            frame "SI 0 Deserializer" {
              n377 = xnode "FPGA I/O Node"("I/O Item"=w872, "FPGA I/O In"=refnum<k21> "IO Socket\\SI 0 Deserializer MFP 0 Output Enable") -> ()  [unwired: 1 out]
              n378 = xnode "FPGA I/O Node"("I/O Item"=w871, "FPGA I/O In"=refnum<k21> "IO Socket\\SI 0 Deserializer MFP 1 Output Enable") -> ()  [unwired: 1 out]
              n379 = xnode "FPGA I/O Node"("I/O Item"=w870, "FPGA I/O In"=refnum<k21> "IO Socket\\SI 0 Deserializer MFP 4 Output Enable") -> ()  [unwired: 1 out]
              n380 = xnode "FPGA I/O Node"("I/O Item"=w869, "FPGA I/O In"=refnum<k21> "IO Socket\\SI 0 Deserializer MFP 5 Output Enable") -> ()  [unwired: 1 out]
              n381 = xnode "FPGA I/O Node"("I/O Item"=w868, "FPGA I/O In"=refnum<k21> "IO Socket\\SI 0 Deserializer MFP 6 Output Enable") -> ()  [unwired: 1 out]
              n382 = xnode "FPGA I/O Node"("I/O Item"=w860, "FPGA I/O In"=refnum<k21> "IO Socket\\SI 0 Deserializer MFP 7 Output Enable") -> ()  [unwired: 1 out]
              n383 = xnode "FPGA I/O Node"("I/O Item"=w861, "FPGA I/O In"=refnum<k21> "IO Socket\\SI 0 Deserializer MFP 8 Output Enable") -> ()  [unwired: 1 out]
              n384 = xnode "FPGA I/O Node"("I/O Item"=w862, "FPGA I/O In"=refnum<k21> "IO Socket\\SI 0 Deserializer MFP 9 Output Enable") -> ()  [unwired: 1 out]
              n385 = xnode "FPGA I/O Node"("I/O Item"=w863, "FPGA I/O In"=refnum<k21> "IO Socket\\SI 0 Deserializer MFP 10 Output Enable") -> ()  [unwired: 1 out]
            }
            frame "SI 1 Deserializer" {
              n386 = xnode "FPGA I/O Node"("I/O Item"=w890, "FPGA I/O In"=refnum<k21> "IO Socket\\SI 1 Deserializer MFP 0 Output Enable") -> ()  [unwired: 1 out]
              n387 = xnode "FPGA I/O Node"("I/O Item"=w889, "FPGA I/O In"=refnum<k21> "IO Socket\\SI 1 Deserializer MFP 1 Output Enable") -> ()  [unwired: 1 out]
              n388 = xnode "FPGA I/O Node"("I/O Item"=w888, "FPGA I/O In"=refnum<k21> "IO Socket\\SI 1 Deserializer MFP 4 Output Enable") -> ()  [unwired: 1 out]
              n389 = xnode "FPGA I/O Node"("I/O Item"=w887, "FPGA I/O In"=refnum<k21> "IO Socket\\SI 1 Deserializer MFP 5 Output Enable") -> ()  [unwired: 1 out]
              n390 = xnode "FPGA I/O Node"("I/O Item"=w886, "FPGA I/O In"=refnum<k21> "IO Socket\\SI 1 Deserializer MFP 6 Output Enable") -> ()  [unwired: 1 out]
              n391 = xnode "FPGA I/O Node"("I/O Item"=w878, "FPGA I/O In"=refnum<k21> "IO Socket\\SI 1 Deserializer MFP 7 Output Enable") -> ()  [unwired: 1 out]
              n392 = xnode "FPGA I/O Node"("I/O Item"=w879, "FPGA I/O In"=refnum<k21> "IO Socket\\SI 1 Deserializer MFP 8 Output Enable") -> ()  [unwired: 1 out]
              n393 = xnode "FPGA I/O Node"("I/O Item"=w880, "FPGA I/O In"=refnum<k21> "IO Socket\\SI 1 Deserializer MFP 9 Output Enable") -> ()  [unwired: 1 out]
              n394 = xnode "FPGA I/O Node"("I/O Item"=w881, "FPGA I/O In"=refnum<k21> "IO Socket\\SI 1 Deserializer MFP 10 Output Enable") -> ()  [unwired: 1 out]
            }
            frame "SI 2 Deserializer" {
              n395 = xnode "FPGA I/O Node"("I/O Item"=w908, "FPGA I/O In"=refnum<k21> "IO Socket\\SI 2 Deserializer MFP 0 Output Enable") -> ()  [unwired: 1 out]
              n396 = xnode "FPGA I/O Node"("I/O Item"=w907, "FPGA I/O In"=refnum<k21> "IO Socket\\SI 2 Deserializer MFP 1 Output Enable") -> ()  [unwired: 1 out]
              n397 = xnode "FPGA I/O Node"("I/O Item"=w906, "FPGA I/O In"=refnum<k21> "IO Socket\\SI 2 Deserializer MFP 4 Output Enable") -> ()  [unwired: 1 out]
              n398 = xnode "FPGA I/O Node"("I/O Item"=w905, "FPGA I/O In"=refnum<k21> "IO Socket\\SI 2 Deserializer MFP 5 Output Enable") -> ()  [unwired: 1 out]
              n399 = xnode "FPGA I/O Node"("I/O Item"=w904, "FPGA I/O In"=refnum<k21> "IO Socket\\SI 2 Deserializer MFP 6 Output Enable") -> ()  [unwired: 1 out]
              n400 = xnode "FPGA I/O Node"("I/O Item"=w896, "FPGA I/O In"=refnum<k21> "IO Socket\\SI 2 Deserializer MFP 7 Output Enable") -> ()  [unwired: 1 out]
              n401 = xnode "FPGA I/O Node"("I/O Item"=w897, "FPGA I/O In"=refnum<k21> "IO Socket\\SI 2 Deserializer MFP 8 Output Enable") -> ()  [unwired: 1 out]
              n402 = xnode "FPGA I/O Node"("I/O Item"=w898, "FPGA I/O In"=refnum<k21> "IO Socket\\SI 2 Deserializer MFP 9 Output Enable") -> ()  [unwired: 1 out]
              n403 = xnode "FPGA I/O Node"("I/O Item"=w899, "FPGA I/O In"=refnum<k21> "IO Socket\\SI 2 Deserializer MFP 10 Output Enable") -> ()  [unwired: 1 out]
            }
            frame "SI 3 Deserializer" {
              n404 = xnode "FPGA I/O Node"("I/O Item"=w926, "FPGA I/O In"=refnum<k21> "IO Socket\\SI 3 Deserializer MFP 0 Output Enable") -> ()  [unwired: 1 out]
              n405 = xnode "FPGA I/O Node"("I/O Item"=w925, "FPGA I/O In"=refnum<k21> "IO Socket\\SI 3 Deserializer MFP 1 Output Enable") -> ()  [unwired: 1 out]
              n406 = xnode "FPGA I/O Node"("I/O Item"=w924, "FPGA I/O In"=refnum<k21> "IO Socket\\SI 3 Deserializer MFP 4 Output Enable") -> ()  [unwired: 1 out]
              n407 = xnode "FPGA I/O Node"("I/O Item"=w923, "FPGA I/O In"=refnum<k21> "IO Socket\\SI 3 Deserializer MFP 5 Output Enable") -> ()  [unwired: 1 out]
              n408 = xnode "FPGA I/O Node"("I/O Item"=w922, "FPGA I/O In"=refnum<k21> "IO Socket\\SI 3 Deserializer MFP 6 Output Enable") -> ()  [unwired: 1 out]
              n409 = xnode "FPGA I/O Node"("I/O Item"=w914, "FPGA I/O In"=refnum<k21> "IO Socket\\SI 3 Deserializer MFP 7 Output Enable") -> ()  [unwired: 1 out]
              n410 = xnode "FPGA I/O Node"("I/O Item"=w915, "FPGA I/O In"=refnum<k21> "IO Socket\\SI 3 Deserializer MFP 8 Output Enable") -> ()  [unwired: 1 out]
              n411 = xnode "FPGA I/O Node"("I/O Item"=w916, "FPGA I/O In"=refnum<k21> "IO Socket\\SI 3 Deserializer MFP 9 Output Enable") -> ()  [unwired: 1 out]
              n412 = xnode "FPGA I/O Node"("I/O Item"=w917, "FPGA I/O In"=refnum<k21> "IO Socket\\SI 3 Deserializer MFP 10 Output Enable") -> ()  [unwired: 1 out]
            }
            frame "SO 0 Serializer" {
              n413 = xnode "FPGA I/O Node"("I/O Item"=w941, "FPGA I/O In"=refnum<k21> "IO Socket\\SO 0 Serializer MFP 0 Output Enable") -> ()  [unwired: 1 out]
              n414 = xnode "FPGA I/O Node"("I/O Item"=w940, "FPGA I/O In"=refnum<k21> "IO Socket\\SO 0 Serializer MFP 3 Output Enable") -> ()  [unwired: 1 out]
              n415 = xnode "FPGA I/O Node"("I/O Item"=w936, "FPGA I/O In"=refnum<k21> "IO Socket\\SO 0 Serializer MFP 4 Output Enable") -> ()  [unwired: 1 out]
              n416 = xnode "FPGA I/O Node"("I/O Item"=w935, "FPGA I/O In"=refnum<k21> "IO Socket\\SO 0 Serializer MFP 6 Output Enable") -> ()  [unwired: 1 out]
              n417 = xnode "FPGA I/O Node"("I/O Item"=w934, "FPGA I/O In"=refnum<k21> "IO Socket\\SO 0 Serializer MFP 7 Output Enable") -> ()  [unwired: 1 out]
              n418 = xnode "FPGA I/O Node"("I/O Item"=w932, "FPGA I/O In"=refnum<k21> "IO Socket\\SO 0 Serializer MFP 8 Output Enable") -> ()  [unwired: 1 out]
            }
            frame "SO 1 Serializer" {
              n419 = xnode "FPGA I/O Node"("I/O Item"=w953, "FPGA I/O In"=refnum<k21> "IO Socket\\SO 1 Serializer MFP 0 Output Enable") -> ()  [unwired: 1 out]
              n420 = xnode "FPGA I/O Node"("I/O Item"=w952, "FPGA I/O In"=refnum<k21> "IO Socket\\SO 1 Serializer MFP 3 Output Enable") -> ()  [unwired: 1 out]
              n421 = xnode "FPGA I/O Node"("I/O Item"=w948, "FPGA I/O In"=refnum<k21> "IO Socket\\SO 1 Serializer MFP 4 Output Enable") -> ()  [unwired: 1 out]
              n422 = xnode "FPGA I/O Node"("I/O Item"=w947, "FPGA I/O In"=refnum<k21> "IO Socket\\SO 1 Serializer MFP 6 Output Enable") -> ()  [unwired: 1 out]
              n423 = xnode "FPGA I/O Node"("I/O Item"=w946, "FPGA I/O In"=refnum<k21> "IO Socket\\SO 1 Serializer MFP 7 Output Enable") -> ()  [unwired: 1 out]
              n424 = xnode "FPGA I/O Node"("I/O Item"=w944, "FPGA I/O In"=refnum<k21> "IO Socket\\SO 1 Serializer MFP 8 Output Enable") -> ()  [unwired: 1 out]
            }
            frame "SO 2 Serializer" {
              n425 = xnode "FPGA I/O Node"("I/O Item"=w965, "FPGA I/O In"=refnum<k21> "IO Socket\\SO 2 Serializer MFP 0 Output Enable") -> ()  [unwired: 1 out]
              n426 = xnode "FPGA I/O Node"("I/O Item"=w964, "FPGA I/O In"=refnum<k21> "IO Socket\\SO 2 Serializer MFP 3 Output Enable") -> ()  [unwired: 1 out]
              n427 = xnode "FPGA I/O Node"("I/O Item"=w960, "FPGA I/O In"=refnum<k21> "IO Socket\\SO 2 Serializer MFP 4 Output Enable") -> ()  [unwired: 1 out]
              n428 = xnode "FPGA I/O Node"("I/O Item"=w959, "FPGA I/O In"=refnum<k21> "IO Socket\\SO 2 Serializer MFP 6 Output Enable") -> ()  [unwired: 1 out]
              n429 = xnode "FPGA I/O Node"("I/O Item"=w958, "FPGA I/O In"=refnum<k21> "IO Socket\\SO 2 Serializer MFP 7 Output Enable") -> ()  [unwired: 1 out]
              n430 = xnode "FPGA I/O Node"("I/O Item"=w956, "FPGA I/O In"=refnum<k21> "IO Socket\\SO 2 Serializer MFP 8 Output Enable") -> ()  [unwired: 1 out]
            }
            frame "SO 3 Serializer" {
              n431 = xnode "FPGA I/O Node"("I/O Item"=w977, "FPGA I/O In"=refnum<k21> "IO Socket\\SO 3 Serializer MFP 0 Output Enable") -> ()  [unwired: 1 out]
              n432 = xnode "FPGA I/O Node"("I/O Item"=w976, "FPGA I/O In"=refnum<k21> "IO Socket\\SO 3 Serializer MFP 3 Output Enable") -> ()  [unwired: 1 out]
              n433 = xnode "FPGA I/O Node"("I/O Item"=w972, "FPGA I/O In"=refnum<k21> "IO Socket\\SO 3 Serializer MFP 4 Output Enable") -> ()  [unwired: 1 out]
              n434 = xnode "FPGA I/O Node"("I/O Item"=w971, "FPGA I/O In"=refnum<k21> "IO Socket\\SO 3 Serializer MFP 6 Output Enable") -> ()  [unwired: 1 out]
              n435 = xnode "FPGA I/O Node"("I/O Item"=w970, "FPGA I/O In"=refnum<k21> "IO Socket\\SO 3 Serializer MFP 7 Output Enable") -> ()  [unwired: 1 out]
              n436 = xnode "FPGA I/O Node"("I/O Item"=w968, "FPGA I/O In"=refnum<k21> "IO Socket\\SO 3 Serializer MFP 8 Output Enable") -> ()  [unwired: 1 out]
            }
          }
          n437 = Not(x=w850) -> (.not. x?=w849:bool)
        }
        frame condition #10 {
          n438 = case shown="\"SO 1 Serializer\"" w993 {
            tunnel: w992 -> [_ w1007 w1025 w1040 w1052]
            tunnel: w991 -> [_ w1006 w1024 _ _]
            tunnel: w990 -> [_ _ _ _ _]
            tunnel: w989 -> [_ _ _ w1039 w1051]
            tunnel: w988 -> [_ w1005 w1023 w1035 w1047]
            tunnel: w987 -> [_ w1004 w1022 _ _]
            tunnel: w986 -> [_ w1003 w1021 w1034 w1046]
            tunnel: [w994 _ _ _ _] -> w985
            tunnel: w983 -> [_ w995 w1013 w1033 w1045]
            tunnel: w982 -> [_ w996 w1014 w1031 w1043]
            tunnel: w981 -> [_ w997 w1015 _ _]
            tunnel: w980 -> [_ w998 w1016 _ _]
            frame Default {
              w994 = TRUE  # serdes id invalid
            }
            frame "SI 0 Deserializer" {
              n439 = xnode "FPGA I/O Node"("I/O Item"=w1007, "FPGA I/O In"=refnum<k21> "IO Socket\\SI 0 Deserializer MFP 0 Output Enable") -> ()  [unwired: 1 out]
              n440 = xnode "FPGA I/O Node"("I/O Item"=w1006, "FPGA I/O In"=refnum<k21> "IO Socket\\SI 0 Deserializer MFP 1 Output Enable") -> ()  [unwired: 1 out]
              n441 = xnode "FPGA I/O Node"("I/O Item"=w1005, "FPGA I/O In"=refnum<k21> "IO Socket\\SI 0 Deserializer MFP 4 Output Enable") -> ()  [unwired: 1 out]
              n442 = xnode "FPGA I/O Node"("I/O Item"=w1004, "FPGA I/O In"=refnum<k21> "IO Socket\\SI 0 Deserializer MFP 5 Output Enable") -> ()  [unwired: 1 out]
              n443 = xnode "FPGA I/O Node"("I/O Item"=w1003, "FPGA I/O In"=refnum<k21> "IO Socket\\SI 0 Deserializer MFP 6 Output Enable") -> ()  [unwired: 1 out]
              n444 = xnode "FPGA I/O Node"("I/O Item"=w995, "FPGA I/O In"=refnum<k21> "IO Socket\\SI 0 Deserializer MFP 7 Output Enable") -> ()  [unwired: 1 out]
              n445 = xnode "FPGA I/O Node"("I/O Item"=w996, "FPGA I/O In"=refnum<k21> "IO Socket\\SI 0 Deserializer MFP 8 Output Enable") -> ()  [unwired: 1 out]
              n446 = xnode "FPGA I/O Node"("I/O Item"=w997, "FPGA I/O In"=refnum<k21> "IO Socket\\SI 0 Deserializer MFP 9 Output Enable") -> ()  [unwired: 1 out]
              n447 = xnode "FPGA I/O Node"("I/O Item"=w998, "FPGA I/O In"=refnum<k21> "IO Socket\\SI 0 Deserializer MFP 10 Output Enable") -> ()  [unwired: 1 out]
            }
            frame "SI 1 Deserializer" {
              n448 = xnode "FPGA I/O Node"("I/O Item"=w1025, "FPGA I/O In"=refnum<k21> "IO Socket\\SI 1 Deserializer MFP 0 Output Enable") -> ()  [unwired: 1 out]
              n449 = xnode "FPGA I/O Node"("I/O Item"=w1024, "FPGA I/O In"=refnum<k21> "IO Socket\\SI 1 Deserializer MFP 1 Output Enable") -> ()  [unwired: 1 out]
              n450 = xnode "FPGA I/O Node"("I/O Item"=w1023, "FPGA I/O In"=refnum<k21> "IO Socket\\SI 1 Deserializer MFP 4 Output Enable") -> ()  [unwired: 1 out]
              n451 = xnode "FPGA I/O Node"("I/O Item"=w1022, "FPGA I/O In"=refnum<k21> "IO Socket\\SI 1 Deserializer MFP 5 Output Enable") -> ()  [unwired: 1 out]
              n452 = xnode "FPGA I/O Node"("I/O Item"=w1021, "FPGA I/O In"=refnum<k21> "IO Socket\\SI 1 Deserializer MFP 6 Output Enable") -> ()  [unwired: 1 out]
              n453 = xnode "FPGA I/O Node"("I/O Item"=w1013, "FPGA I/O In"=refnum<k21> "IO Socket\\SI 1 Deserializer MFP 7 Output Enable") -> ()  [unwired: 1 out]
              n454 = xnode "FPGA I/O Node"("I/O Item"=w1014, "FPGA I/O In"=refnum<k21> "IO Socket\\SI 1 Deserializer MFP 8 Output Enable") -> ()  [unwired: 1 out]
              n455 = xnode "FPGA I/O Node"("I/O Item"=w1015, "FPGA I/O In"=refnum<k21> "IO Socket\\SI 1 Deserializer MFP 9 Output Enable") -> ()  [unwired: 1 out]
              n456 = xnode "FPGA I/O Node"("I/O Item"=w1016, "FPGA I/O In"=refnum<k21> "IO Socket\\SI 1 Deserializer MFP 10 Output Enable") -> ()  [unwired: 1 out]
            }
            frame "SO 0 Serializer" {
              n457 = xnode "FPGA I/O Node"("I/O Item"=w1040, "FPGA I/O In"=refnum<k21> "IO Socket\\SO 0 Serializer MFP 0 Output Enable") -> ()  [unwired: 1 out]
              n458 = xnode "FPGA I/O Node"("I/O Item"=w1039, "FPGA I/O In"=refnum<k21> "IO Socket\\SO 0 Serializer MFP 3 Output Enable") -> ()  [unwired: 1 out]
              n459 = xnode "FPGA I/O Node"("I/O Item"=w1035, "FPGA I/O In"=refnum<k21> "IO Socket\\SO 0 Serializer MFP 4 Output Enable") -> ()  [unwired: 1 out]
              n460 = xnode "FPGA I/O Node"("I/O Item"=w1034, "FPGA I/O In"=refnum<k21> "IO Socket\\SO 0 Serializer MFP 6 Output Enable") -> ()  [unwired: 1 out]
              n461 = xnode "FPGA I/O Node"("I/O Item"=w1033, "FPGA I/O In"=refnum<k21> "IO Socket\\SO 0 Serializer MFP 7 Output Enable") -> ()  [unwired: 1 out]
              n462 = xnode "FPGA I/O Node"("I/O Item"=w1031, "FPGA I/O In"=refnum<k21> "IO Socket\\SO 0 Serializer MFP 8 Output Enable") -> ()  [unwired: 1 out]
            }
            frame "SO 1 Serializer" {
              n463 = xnode "FPGA I/O Node"("I/O Item"=w1052, "FPGA I/O In"=refnum<k21> "IO Socket\\SO 1 Serializer MFP 0 Output Enable") -> ()  [unwired: 1 out]
              n464 = xnode "FPGA I/O Node"("I/O Item"=w1051, "FPGA I/O In"=refnum<k21> "IO Socket\\SO 1 Serializer MFP 3 Output Enable") -> ()  [unwired: 1 out]
              n465 = xnode "FPGA I/O Node"("I/O Item"=w1047, "FPGA I/O In"=refnum<k21> "IO Socket\\SO 1 Serializer MFP 4 Output Enable") -> ()  [unwired: 1 out]
              n466 = xnode "FPGA I/O Node"("I/O Item"=w1046, "FPGA I/O In"=refnum<k21> "IO Socket\\SO 1 Serializer MFP 6 Output Enable") -> ()  [unwired: 1 out]
              n467 = xnode "FPGA I/O Node"("I/O Item"=w1045, "FPGA I/O In"=refnum<k21> "IO Socket\\SO 1 Serializer MFP 7 Output Enable") -> ()  [unwired: 1 out]
              n468 = xnode "FPGA I/O Node"("I/O Item"=w1043, "FPGA I/O In"=refnum<k21> "IO Socket\\SO 1 Serializer MFP 8 Output Enable") -> ()  [unwired: 1 out]
            }
          }
          n469 = Not(x=w985) -> (.not. x?=w984:bool)
        }
        frame condition #11 (active) {
          w1055 = TRUE ("assert")
          # "Target not supported"
          n470 = call <instrlib>:"Assert.vi"("assert"=w1055, "error code"=-1, "enable show error"=w1055) -> ()  [unwired: 13 in]
        }
      }
    }
  }
  "serdes id valid" <- w13
